vi "Settings Dialog.vi"(8 "error in (no error)":errorcluster, 11 "Feed Module Config in":T18={"GUID"="", "Drop Coords"={"Horizontal"=0, "Vertical"=0}, "Process Name"="", "Queue Name"="", "Settings"={"Cycle Period"=500.0, "Ismatech"={"VISA resource name"="", "Simulated?"=TRUE, "Pump Number"=1.0, "Reverse?"=FALSE}, "Masterflex"={"VISA resource name"="", "Simulated?"=TRUE, "Pump Number"=1.0, "Reverse?"=FALSE}, "Mettler"={"VISA resource name"="", "Simulated?"=FALSE}, "Bronkhorst M13 Flow Meter"={"VISA resource name"="", "Simulated?"=TRUE, "Smoothing Steps"=1}, "PID 2 Parameters"={"Input Device"=enum."Default", "Output Device"=enum."Default", "Setpoint"=0.0, "PID gains"={"proportional gain (Kc)"=1.0, "integral time (Ti, min)"=0.01, "derivative time (Td, min)"=0.0}}, "Manual Entry"=0.0, "Auto?"=TRUE, "output range"={"output high"=100.0, "output low"=0.0}, "Tacmina Settings"={"Analog DAQ Task"="", "Digital DAQ Task"=""}, "KNF SIMDOS Settings"={"VISA resource name"="", "Simulated?"=TRUE}, "ASIA Pump C"={"ASIA Pump #"=-1, "channel"=-1, "Simulated"=FALSE}, "VICI Settings"={"VISA resource name"="", "Simulated?"=TRUE, "Pump Letter"="", "Reverse?"=FALSE}, "FLOM Settings"={"VISA resource name"="", "Simulated?"=TRUE, "Pump Number"=0.0}, "SSI PR/LD Settings"={"VISA resource name"="", "Simulated?"=FALSE}, "Masterflex 75211 Settings"={"Analog DAQ Task"="", "Digital DAQ Task"=""}, "SSI P40 Settings"={"VISA resource name"="", "Simulated?"=TRUE}, "Ismatech 3 Channel Settings"={"VISA resource name"="", "Pump Number"=1, "Channel Number"=0, "Simulated?"=TRUE, "Reverse?"=FALSE}, "Bronkhorst M14 Settings"={"VISA resource name"="", "Simulated?"=FALSE, "Smoothing Steps"=1}}, "Settings Load Count"=0, "OP Load Count"=0} {"Settings"."Bronkhorst M14 Settings"."Smoothing Steps" min=1 step=1; "Settings"."Ismatech 3 Channel Settings"."Channel Number" min=0 max=3; "Settings"."Ismatech 3 Channel Settings"."Pump Number" min=1; "Settings"."output range"."output low" min=0.0 max=100.0 format="%.2f"; "Settings"."output range"."output high" format="%.2f"; "Settings"."PID 2 Parameters"."PID gains"."derivative time (Td, min)" format="%.3f"; "Settings"."PID 2 Parameters"."PID gains"."integral time (Ti, min)" format="%.3f"; "Settings"."PID 2 Parameters"."PID gains"."proportional gain (Kc)" format="%.3f"; "Settings"."Bronkhorst M13 Flow Meter"."Smoothing Steps" min=1 step=1; "Settings"."ASIA Pump C"."channel" min=0 max=1 step=1; "Settings"."Ismatech"."Pump Number" min=1.0 max=20.0 step=1.0; "Settings"."Masterflex"."Pump Number" min=1.0 max=20.0 step=1.0}) -> (0 "error out":errorcluster, 1 "Cancelled?":bool=TRUE, 2 "UI Refresh Needed?":bool, 3 "Feed Module Config out":T18={"GUID"="", "Drop Coords"={"Horizontal"=0, "Vertical"=0}, "Process Name"="", "Queue Name"="", "Settings"={"Cycle Period"=500.0, "Ismatech"={"VISA resource name"="", "Simulated?"=TRUE, "Pump Number"=1.0, "Reverse?"=FALSE}, "Masterflex"={"VISA resource name"="", "Simulated?"=TRUE, "Pump Number"=1.0, "Reverse?"=FALSE}, "Mettler"={"VISA resource name"="", "Simulated?"=FALSE}, "Bronkhorst M13 Flow Meter"={"VISA resource name"="", "Simulated?"=TRUE, "Smoothing Steps"=1}, "PID 2 Parameters"={"Input Device"=enum."Default", "Output Device"=enum."Default", "Setpoint"=0.0, "PID gains"={"proportional gain (Kc)"=1.0, "integral time (Ti, min)"=0.01, "derivative time (Td, min)"=0.0}}, "Manual Entry"=0.0, "Auto?"=TRUE, "output range"={"output high"=100.0, "output low"=0.0}, "Tacmina Settings"={"Analog DAQ Task"="", "Digital DAQ Task"=""}, "KNF SIMDOS Settings"={"VISA resource name"="", "Simulated?"=TRUE}, "ASIA Pump C"={"ASIA Pump #"=0, "channel"=0, "Simulated"=FALSE}, "VICI Settings"={"VISA resource name"="", "Simulated?"=TRUE, "Pump Letter"="", "Reverse?"=FALSE}, "FLOM Settings"={"VISA resource name"="", "Simulated?"=TRUE, "Pump Number"=0.0}, "SSI PR/LD Settings"={"VISA resource name"="", "Simulated?"=FALSE}, "Masterflex 75211 Settings"={"Analog DAQ Task"="", "Digital DAQ Task"=""}, "SSI P40 Settings"={"VISA resource name"="", "Simulated?"=TRUE}, "Ismatech 3 Channel Settings"={"VISA resource name"="", "Pump Number"=1, "Channel Number"=0, "Simulated?"=TRUE, "Reverse?"=FALSE}, "Bronkhorst M14 Settings"={"VISA resource name"="", "Simulated?"=FALSE, "Smoothing Steps"=1}}, "Settings Load Count"=0, "OP Load Count"=0} {"Settings"."Bronkhorst M14 Settings"."Smoothing Steps" min=1 step=1; "Settings"."Ismatech 3 Channel Settings"."Channel Number" min=0 max=3; "Settings"."Ismatech 3 Channel Settings"."Pump Number" min=1; "Settings"."output range"."output low" min=0.0 max=100.0 format="%.2f"; "Settings"."output range"."output high" format="%.2f"; "Settings"."PID 2 Parameters"."PID gains"."derivative time (Td, min)" format="%.3f"; "Settings"."PID 2 Parameters"."PID gains"."integral time (Ti, min)" format="%.3f"; "Settings"."PID 2 Parameters"."PID gains"."proportional gain (Kc)" format="%.3f"; "Settings"."Bronkhorst M13 Flow Meter"."Smoothing Steps" min=1 step=1; "Settings"."ASIA Pump C"."channel" min=0 max=1 step=1; "Settings"."Ismatech"."Pump Number" min=1.0 max=20.0 step=1.0; "Settings"."Masterflex"."Pump Number" min=1.0 max=20.0 step=1.0})   [LabVIEW 2018, in "Feed Module.lvlib" / "Settings.lvlib"]
doc: "Dialog for selecting user specified settings."
uses:
  Settings.lvlib
  Feed Module/Controls/Feed Module Config Cluster.ctl
  <vilib>/Utility/miscctls.llb/LVPoint32TypeDef.ctl
  Feed Module/Controls/Feed Module Settings Cluster.ctl
  Ismatec ISM 831C/Controls/Ismatech ISM831C Settings Cluster.ctl
  Masterflex 7550-30/Controls/Settings Cluster.ctl
  Mettler Toledo/Controls/Settings Cluster.ctl
  Bronkhorst M13 Flow Meter/Settings Cluster.ctl
  Measure Instrument/PID 2 Parameters Cluster.ctl
  Measure Instrument/PID Input Enum.ctl
  Measure Instrument/PID 2 Output Enum.ctl
  Tacmina QI/Tacmina QI DAQ Setting.ctl
  KNF Pump/Settings Cluster plus SIMDOS.ctl
  ASIA Pump/Pump Settings.ctl
  VICI M50 Party Mode/Settings Cluster.ctl
  FLOM Pump/Settings Cluster.ctl
  SSI PR Class/SSI PR or LD Settings Cluster.ctl
  Masterflex 75211/Masterflex 75211 DAQ Setting.ctl
  SSI PR Class/SSI P40 Settings Cluster.ctl
  Ismatec 78001/Ismatec 4083.ctl
  Bronkhorst M14 Flow Meter/Settings Cluster.ctl
  Ismatec ISM 831C/Ismatec ISM 831C.lvlib
  Masterflex 7550-30/Masterflex 7550-30.lvlib
  Mettler Toledo/Mettler Toledo.lvlib
  Bronkhorst M13 Flow Meter/Bronkhorst M13 Flow Meter.lvlib
  Bronkhorst M14 Flow Meter/Bronkhorst M14 Flow Meter.lvlib
  KNF Pump/KNF SIMDOS.lvlib
  VICI M50 Party Mode/VICI M6 M50 Party Mode.lvlib
  FLOM Pump/FLOM Pump.lvlib
  ASIA Pump.lvlib
  SSI PR Class/SSI PR or LD Pump.lvlib
  SSI PR Class/SSI P40 Pump.lvlib
  Ismatec 78001/Ismatec 4308.lvlib
  Feed Module/Feed Module.lvlib
  Tacmina QI/Tacmina QI.lvlib
  Masterflex 75211/Masterflex 75211.lvlib
panel:
  in  "Module Name":string
  in  "Settings Dialog":T17={"Cycle Period"=500.0, "Ismatech"={"VISA resource name"="", "Simulated?"=FALSE, "Pump Number"=1.0, "Reverse?"=FALSE}, "Masterflex"={"VISA resource name"="", "Simulated?"=FALSE, "Pump Number"=1.0, "Reverse?"=FALSE}, "Mettler"={"VISA resource name"="", "Simulated?"=FALSE}, "Bronkhorst M13 Settings"={"VISA resource name"="", "Simulated?"=FALSE, "Smoothing Steps"=1}, "PID 2 Parameters"={"Input Device"=enum."Default", "Output Device"=enum."Default", "PID gains"={"proportional gain (Kc)"=1.0, "integral time (Ti, min)"=0.01, "derivative time (Td, min)"=0.0}}, "PID2 Range"={"output high"=100.0, "output low"=0.0}, "Bronkhorst M14 Settings"={"VISA resource name"="", "Simulated?"=FALSE, "Smoothing Steps"=1}, "Tacmina Settings"={"Analog DAQ Task"="", "Digital DAQ Task"=""}, "KNF SIMDOS Settings"={"VISA resource name"="", "Simulated?"=FALSE}, "ASIA Pump C"={"ASIA Pump #"=-1, "channel"=-1, "Simulated"=FALSE}, "VICI M50 Settings"={"VISA resource name"="", "Simulated?"=FALSE, "Pump Letter"="", "Reverse?"=FALSE}, "FLOM Settings"={"VISA resource name"="", "Simulated?"=FALSE, "Pump Number"=1.0}, "SSI PR/LD Settings"={"VISA resource name"="", "Simulated?"=FALSE}, "Masterflex 75211 Settings"={"Analog DAQ Task"="", "Digital DAQ Task"=""}, "SSI P40 Settings"={"VISA resource name"="", "Simulated?"=FALSE}, "Ismatech 3 Channel Settings"={"VISA resource name"="", "Pump Number"=0, "Channel Number"=0, "Simulated?"=FALSE, "Reverse?"=FALSE}} {"Ismatech 3 Channel Settings"."Channel Number" min=0 max=3; "Ismatech 3 Channel Settings"."Pump Number" min=1; "ASIA Pump C"."channel" min=-1 max=1 step=1; "Bronkhorst M14 Settings"."Smoothing Steps" min=1 step=1; "PID2 Range"."output low" min=0.0 max=100.0 format="%.2f"; "PID2 Range"."output high" format="%.2f"; "PID 2 Parameters"."PID gains"."derivative time (Td, min)" format="%.3f"; "PID 2 Parameters"."PID gains"."integral time (Ti, min)" format="%.3f"; "PID 2 Parameters"."PID gains"."proportional gain (Kc)" format="%.3f"; "Bronkhorst M13 Settings"."Smoothing Steps" min=1 step=1; "Masterflex"."Pump Number" min=1.0 max=20.0 step=1.0; "Ismatech"."Pump Number" min=1.0 max=20.0 step=1.0}
  in  "Cancel Button":bool
  in  "OK Button":bool
  # "Non visible portion of dialog (needed for connector pane)."
  # "Output Instruments"
  # "Input Instruments"
  # "Output Instruments"
  # "Input Instruments"
  # "Output Instruments"
  # "Input Instruments"
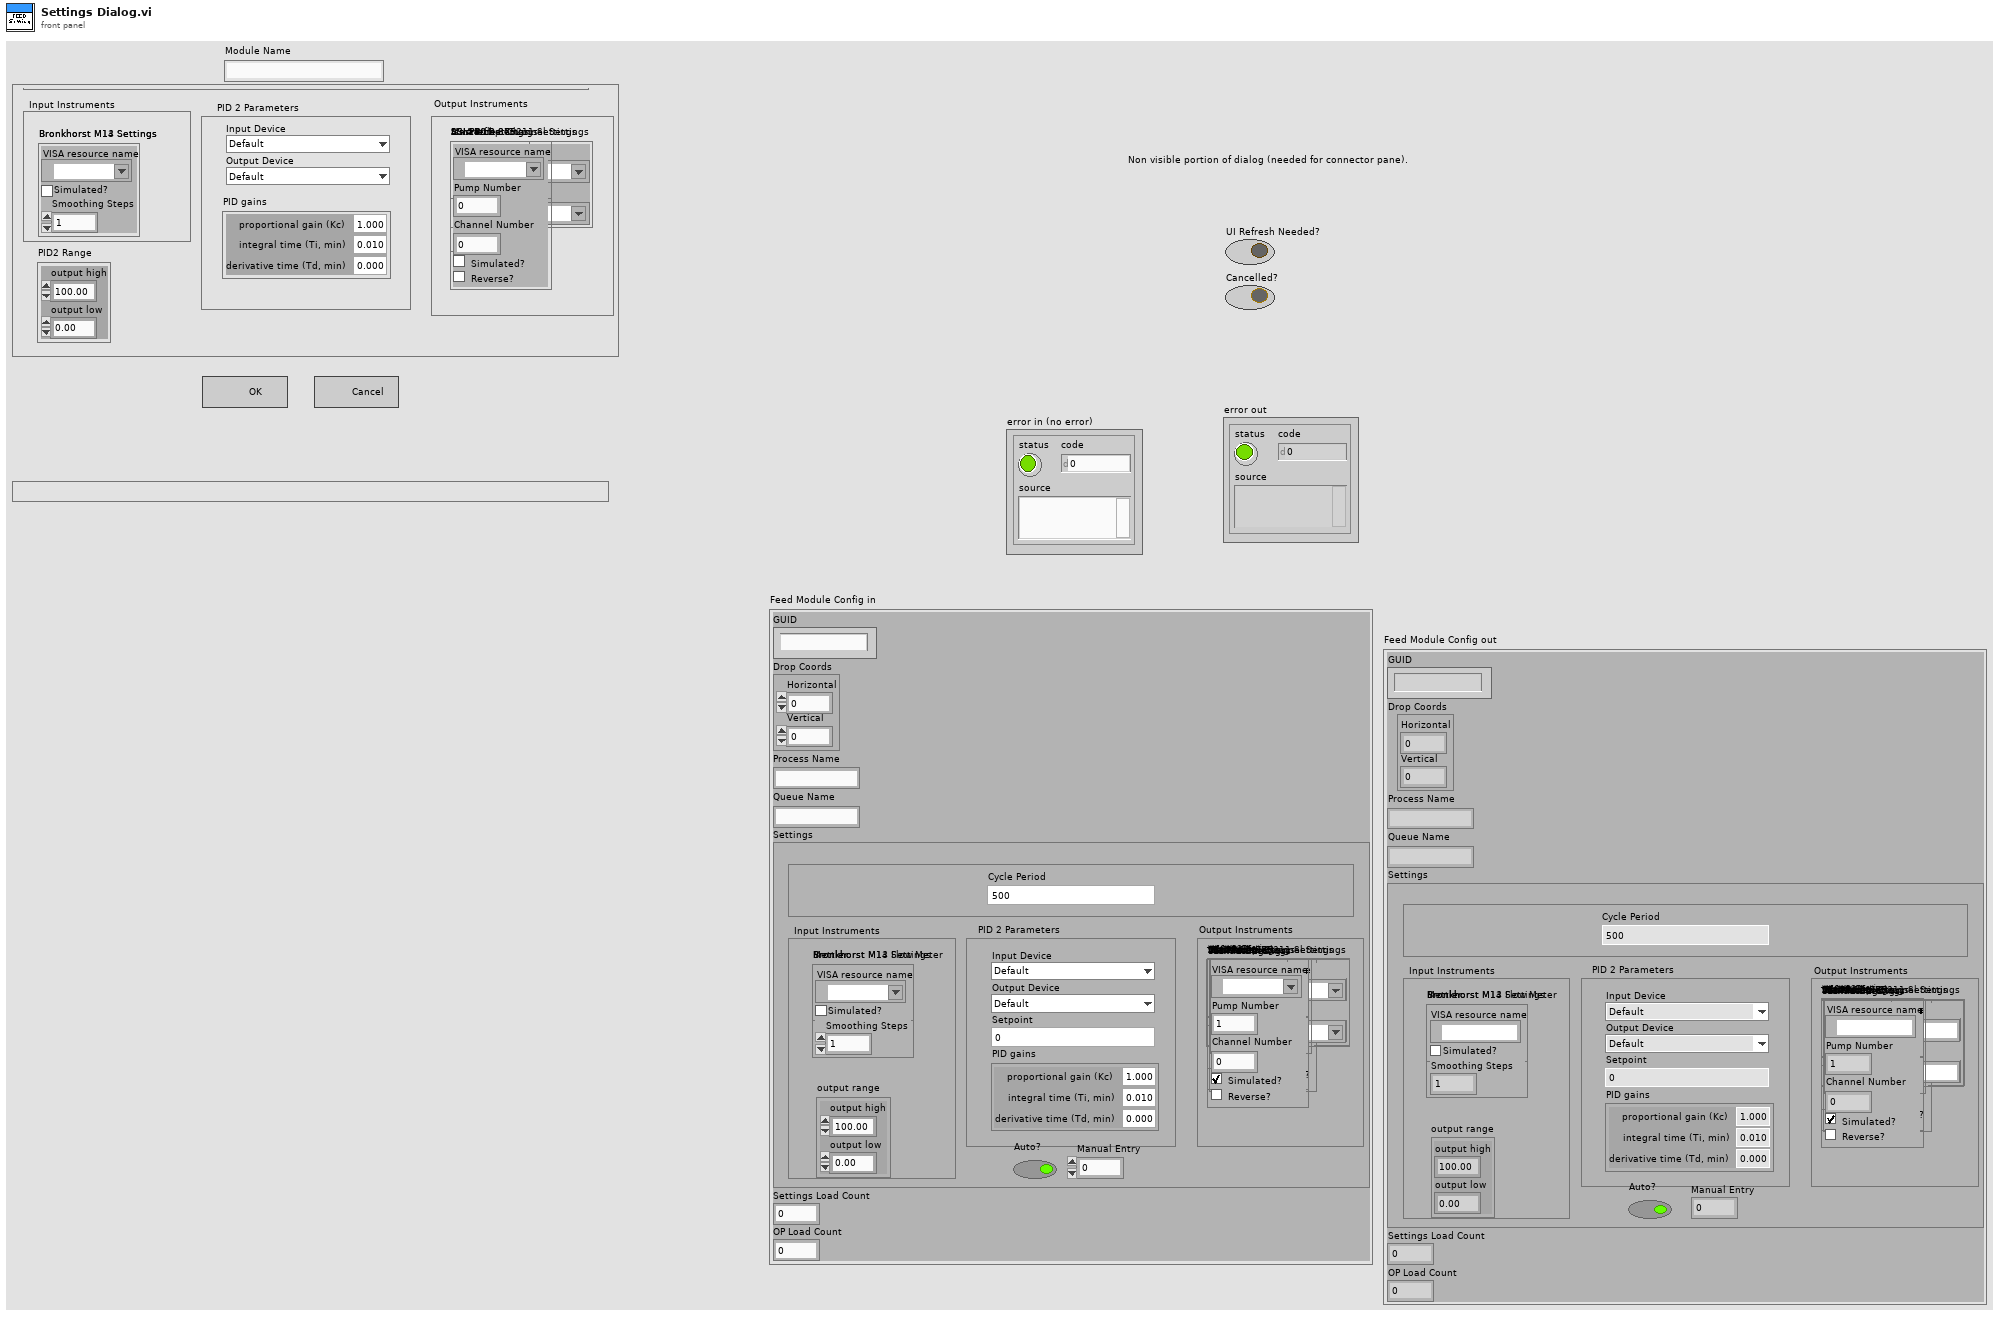
[diagram p1: front panel]
types:
  T1 = typedef "Ismatec ISM 831C.lvlib/Ismatech ISM831C Settings Cluster.ctl" = cluster{"VISA resource name":refnum<visa-resource-name>, "Simulated?":bool, "Pump Number":dbl, "Reverse?":bool}
  T2 = typedef "Masterflex 7550-30.lvlib/Settings Cluster.ctl" = cluster{"VISA resource name":refnum<visa-resource-name>, "Simulated?":bool, "Pump Number":dbl, "Reverse?":bool}
  T3 = typedef "Mettler Toledo.lvlib/Settings Cluster.ctl" = cluster{"VISA resource name":refnum<visa-resource-name>, "Simulated?":bool}
  T4 = typedef "Bronkhorst M13 Flow Meter.lvlib/Settings Cluster.ctl" = cluster{"VISA resource name":refnum<visa-resource-name>, "Simulated?":bool, "Smoothing Steps":i32}
  T5 = typedef "PID Input Enum.ctl" = enum16{"Default", "Bronkhorst M13", "Bronkhorst M14", "Scale Rate of Change"}
  T6 = typedef "PID 2 Output Enum.ctl" = enum16{"Default", "Ismatec ISM 4308", "Ismatec ISM 831C", "Masterflex 7550-30", "VICI", "Tacmina QI", "KNF SIMDOS", "ASIA Type C", "FLOM UI-22-11", "SSI PR/LD", "SSI P40", "Masterflex 75211-70"}
  T7 = typedef "Bronkhorst M14 Flow Meter.lvlib/Settings Cluster.ctl" = cluster{"VISA resource name":refnum<visa-resource-name>, "Simulated?":bool, "Smoothing Steps":i32}
  T8 = typedef "Tacmina QI.lvlib/Tacmina QI DAQ Setting.ctl" = cluster{"Analog DAQ Task":refnum<k21>, "Digital DAQ Task":refnum<k21>}
  T9 = typedef "KNF SIMDOS.lvlib/Settings Cluster plus SIMDOS.ctl" = cluster{"VISA resource name":refnum<visa-resource-name>, "Simulated?":bool}
  T10 = typedef "ASIA Pump.lvlib/Pump Settings.ctl" = cluster{"ASIA Pump #":i32, "channel":i32, "Simulated":bool}
  T11 = typedef "VICI M6 M50 Party Mode.lvlib/Settings Cluster.ctl" = cluster{"VISA resource name":refnum<visa-resource-name>, "Simulated?":bool, "Pump Letter":string, "Reverse?":bool}
  T12 = typedef "FLOM Pump.lvlib/Settings Cluster.ctl" = cluster{"VISA resource name":refnum<visa-resource-name>, "Simulated?":bool, "Pump Number":dbl}
  T13 = typedef "SSI PR or LD Pump.lvlib/SSI PR or LD Settings Cluster.ctl" = cluster{"VISA resource name":refnum<visa-resource-name>, "Simulated?":bool}
  T14 = typedef "Masterflex 75211.lvlib/Masterflex 75211 DAQ Setting.ctl" = cluster{"Analog DAQ Task":refnum<k21>, "Digital DAQ Task":refnum<k21>}
  T15 = typedef "SSI P40 Pump.lvlib/SSI P40 Settings Cluster.ctl" = cluster{"VISA resource name":refnum<visa-resource-name>, "Simulated?":bool}
  T16 = typedef "Ismatec 4308.lvlib/Ismatec 4083.ctl" = cluster{"VISA resource name":refnum<visa-resource-name>, "Pump Number":i16, "Channel Number":i16, "Simulated?":bool, "Reverse?":bool}
  T17 = cluster{"Cycle Period":dbl, "Ismatech":T1, "Masterflex":T2, "Mettler":T3, "Bronkhorst M13 Settings":T4, "PID 2 Parameters":cluster{"Input Device":T5, "Output Device":T6, "PID gains":cluster{"proportional gain (Kc)":dbl, "integral time (Ti, min)":dbl, "derivative time (Td, min)":dbl}}, "PID2 Range":cluster{"output high":dbl, "output low":dbl}, "Bronkhorst M14 Settings":T7, "Tacmina Settings":T8, "KNF SIMDOS Settings":T9, "ASIA Pump C":T10, "VICI M50 Settings":T11, "FLOM Settings":T12, "SSI PR/LD Settings":T13, "Masterflex 75211 Settings":T14, "SSI P40 Settings":T15, "Ismatech 3 Channel Settings":T16}
  T18 = typedef "Feed Module.lvlib/Feed Module Config Cluster.ctl" = cluster{"GUID":string, "Drop Coords":T19, "Process Name":string, "Queue Name":string, "Settings":T20, "Settings Load Count":i32, "OP Load Count":i32}
  T19 = typedef "LVPoint32TypeDef.ctl" = cluster{"Horizontal":i32, "Vertical":i32}
  T20 = typedef "Feed Module.lvlib/Feed Module Settings Cluster.ctl" = cluster{"Cycle Period":dbl, "Ismatech":T1, "Masterflex":T2, "Mettler":T3, "Bronkhorst M13 Flow Meter":T4, "PID 2 Parameters":T21, "Manual Entry":dbl, "Auto?":bool, "output range":cluster{"output high":dbl, "output low":dbl}, "Tacmina Settings":T8, "KNF SIMDOS Settings":T9, "ASIA Pump C":T10, "VICI Settings":T11, "FLOM Settings":T12, "SSI PR/LD Settings":T13, "Masterflex 75211 Settings":T14, "SSI P40 Settings":T15, "Ismatech 3 Channel Settings":T16, "Bronkhorst M14 Settings":T7}
  T21 = typedef "PID 2 Parameters Cluster.ctl" = cluster{"Input Device":T5, "Output Device":T6, "Setpoint":dbl, "PID gains":cluster{"proportional gain (Kc)":dbl, "integral time (Ti, min)":dbl, "derivative time (Td, min)":dbl}}
  T22 = enum8{"Enabled", "Disabled", "Disabled and Grayed Out"}
  T23 = cluster{"Input Device":T5, "Output Device":T6, "PID gains":cluster{"proportional gain (Kc)":dbl, "integral time (Ti, min)":dbl, "derivative time (Td, min)":dbl}}
  T24 = cluster{"proportional gain (Kc)":dbl, "integral time (Ti, min)":dbl, "derivative time (Td, min)":dbl}
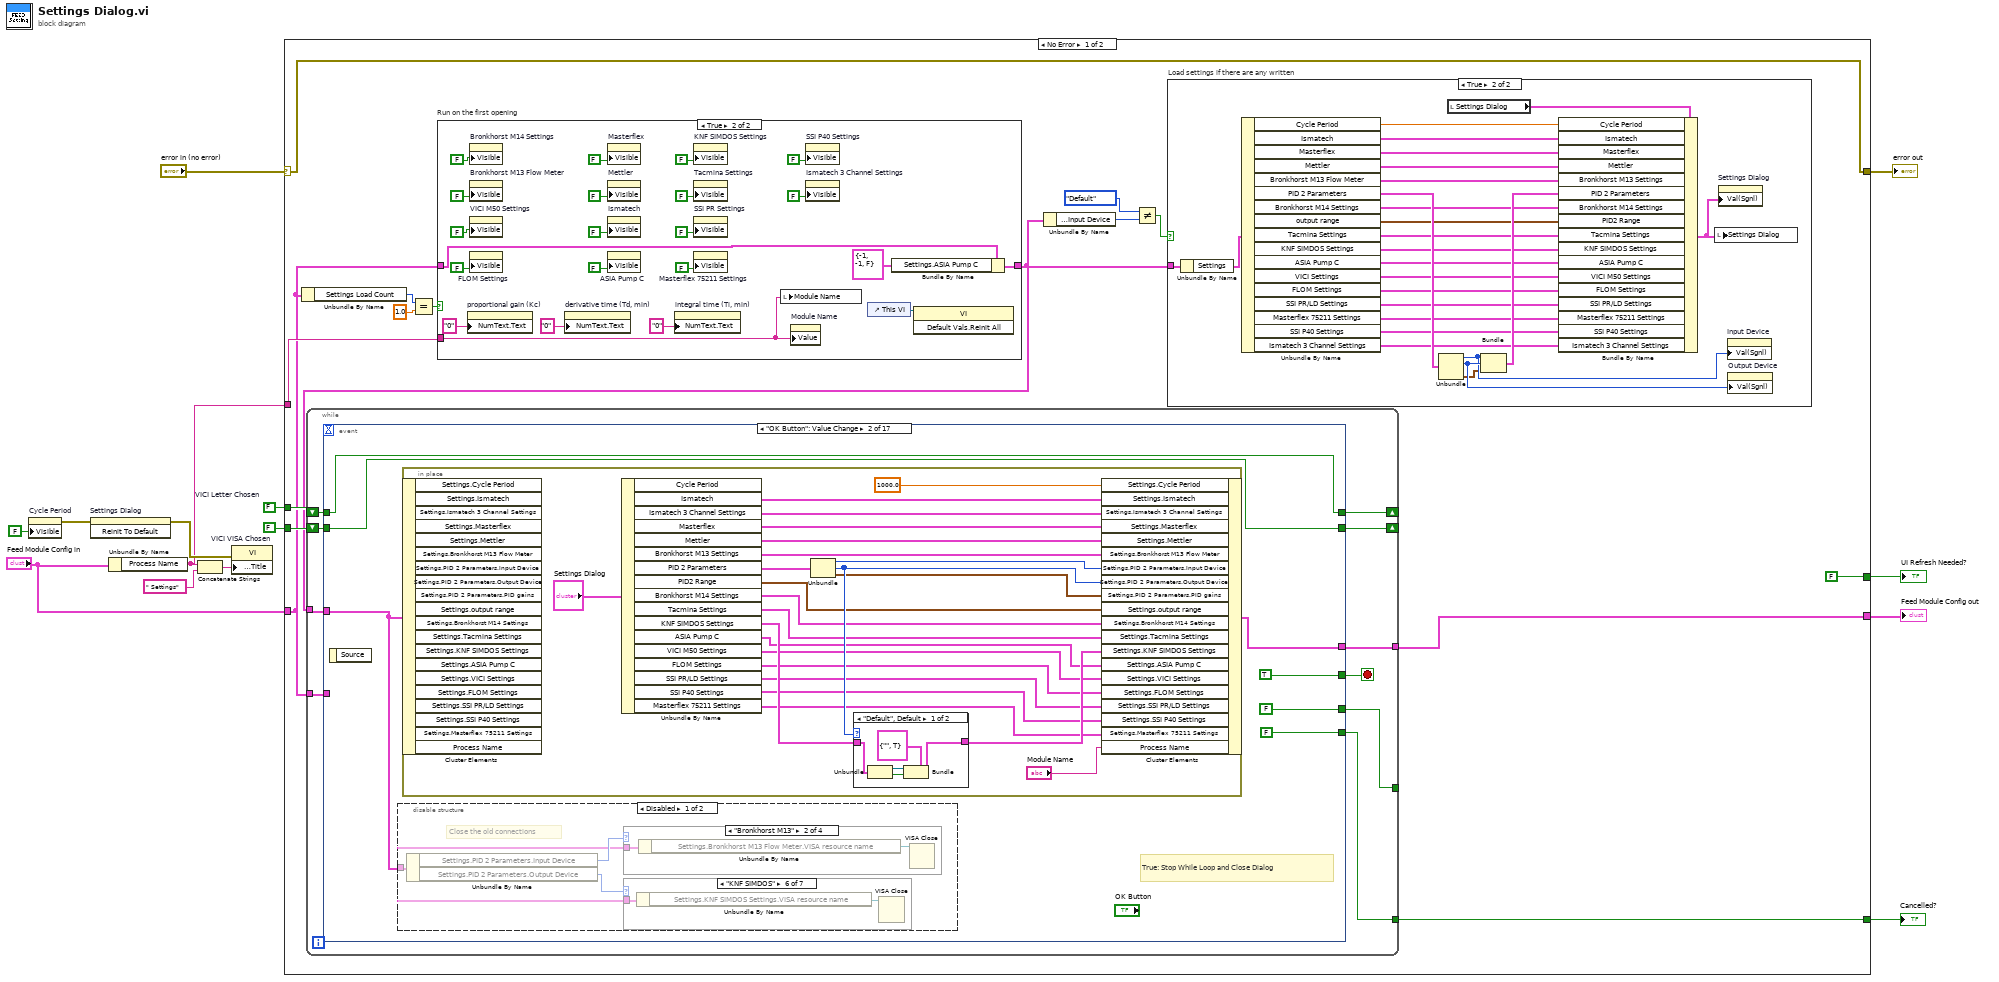
[diagram p0: block diagram]
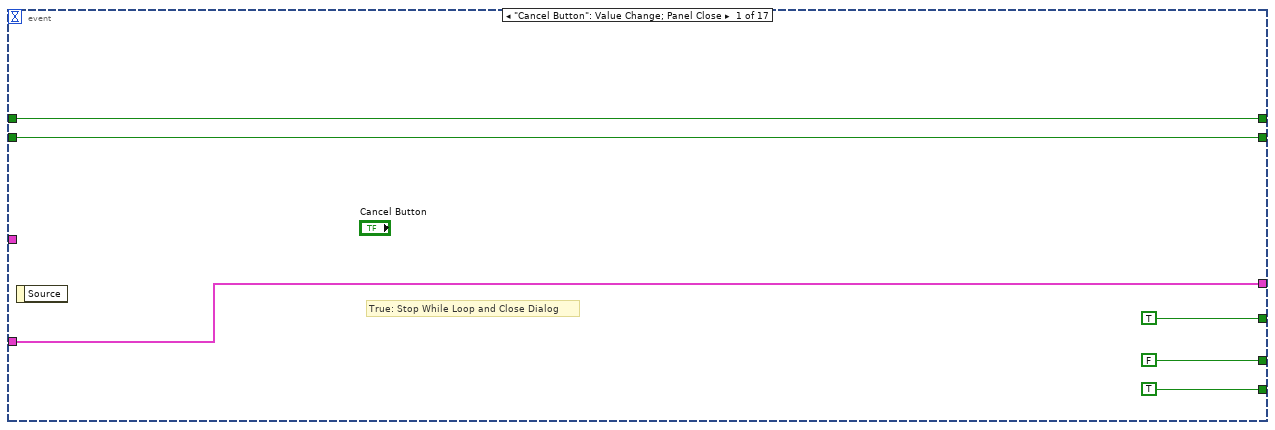
[diagram p4: hidden frame]
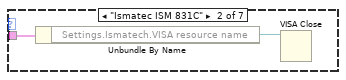
[diagram p6: hidden frame]
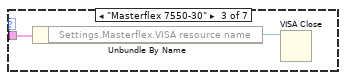
[diagram p7: hidden frame]
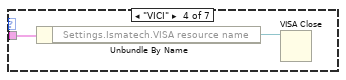
[diagram p8: hidden frame]
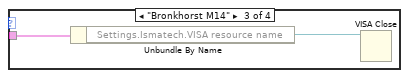
[diagram p12: hidden frame]
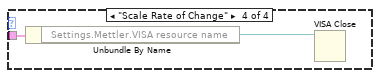
[diagram p13: hidden frame]
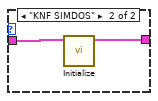
[diagram p15: hidden frame]
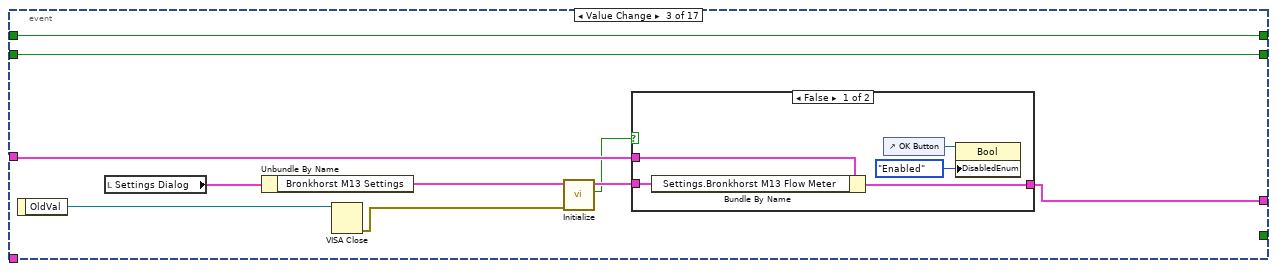
[diagram p16: hidden frame]
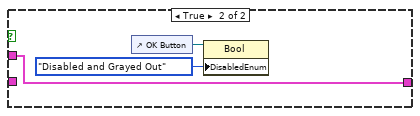
[diagram p17: hidden frame]
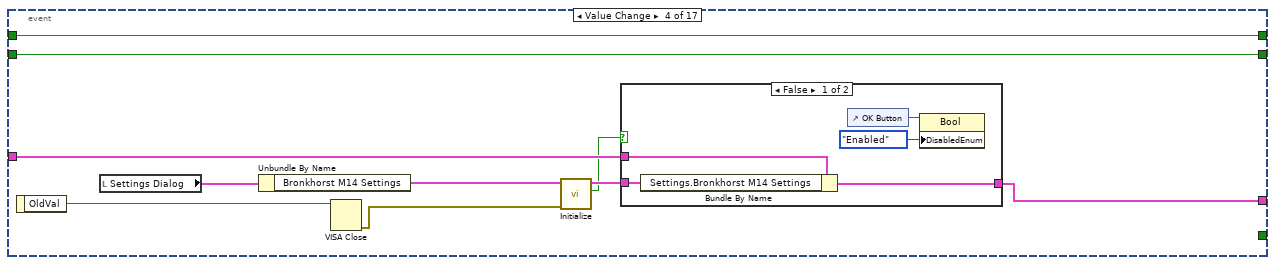
[diagram p18: hidden frame]
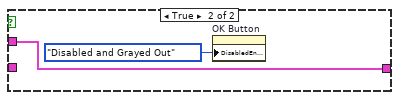
[diagram p19: hidden frame]
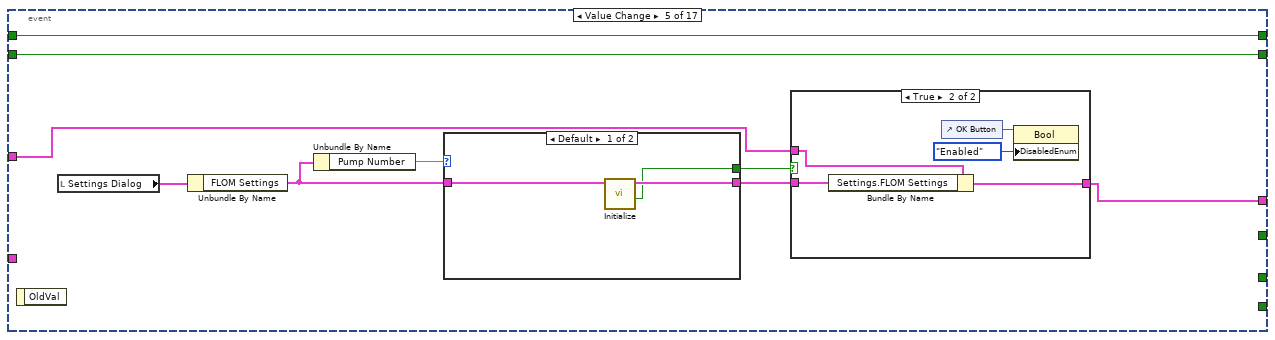
[diagram p20: hidden frame]
diagram:
  w5 = FALSE  # VICI VISA Chosen
  w6 = FALSE  # VICI Letter Chosen
  n1 = property on="Cycle Period" class="DigNum (strict)"("Visible"=FALSE) -> (error out=w3:errorcluster)  [unwired: 2 in, 1 out]
  n2 = invoke on="Settings Dialog" class="Clust (strict)" method="Reinit To Default"(error in=w3) -> (error out=w2:errorcluster)  [unwired: 2 in, 2 out]
  n3 = Unbundle By Name("Feed Module Config in") -> ("Process Name"=w1:string)
  n4 = Concatenate Strings(w1, " Settings" ("string")) -> (w8:string)
  n5 = property class="VI"(error in=w2, "Front Panel.Title"=w8) -> ()  [unwired: 1 in, 2 out]
  n6 = case shown="No Error" "error in (no error)" {
    selector: "error in (no error)" -> [w29 w630]
    tunnel: [w29 w630] -> w14
    tunnel: "Feed Module Config in" -> [w15 w629]
    tunnel: [w27 w629] -> w10
    tunnel: [FALSE ("UI Refresh Needed?") _] -> w13
    tunnel: [w26 TRUE ("UI Refresh Needed?")] -> w12
    tunnel: w6 -> [w22 _]
    tunnel: w5 -> [w21 _]
    tunnel: w1 -> [w20 _]
    frame No Error {
      n7 = Unbundle By Name(w15) -> ("Settings Load Count"=w25:i32)
      n8 = Equal?(x=w25, y=1.0) -> (x = y?=w23:bool)
      n9 = case "Run on the first opening" shown="True" w23 {
        tunnel: w15 -> [w55 w64]
        tunnel: [w55 w63] -> w19
        tunnel: w20 -> [_ w60]
        frame False {
        }
        frame True {
          n10 = property on="proportional gain (Kc)" class="DigNum (strict)"("NumText.Text"="0" ("Numeric Text.Text")) -> ()  [unwired: 2 in, 2 out]
          n11 = property on="Bronkhorst M14 Settings" class="Clust (strict)"("Visible"=FALSE) -> ()  [unwired: 2 in, 2 out]
          n12 = property on="Bronkhorst M13 Flow Meter" class="Clust (strict)"("Visible"=FALSE) -> ()  [unwired: 2 in, 2 out]
          n13 = property on="VICI M50 Settings" class="Clust (strict)"("Visible"=FALSE) -> ()  [unwired: 2 in, 2 out]
          n14 = property on="FLOM Settings" class="Clust (strict)"("Visible"=FALSE) -> ()  [unwired: 2 in, 2 out]
          n15 = property on="derivative time (Td, min)" class="DigNum (strict)"("NumText.Text"="0" ("Numeric Text.Text")) -> ()  [unwired: 2 in, 2 out]
          n16 = property on="Masterflex" class="Clust (strict)"("Visible"=FALSE) -> ()  [unwired: 2 in, 2 out]
          n17 = property on="Mettler" class="Clust (strict)"("Visible"=FALSE) -> ()  [unwired: 2 in, 2 out]
          n18 = property on="Ismatech" class="Clust (strict)"("Visible"=FALSE) -> ()  [unwired: 2 in, 2 out]
          n19 = property on="ASIA Pump C" class="Clust (strict)"("Visible"=FALSE) -> ()  [unwired: 2 in, 2 out]
          n20 = property on="integral time (Ti, min)" class="DigNum (strict)"("NumText.Text"="0" ("Numeric Text.Text")) -> ()  [unwired: 2 in, 2 out]
          n21 = property on="KNF SIMDOS Settings" class="Clust (strict)"("Visible"=FALSE) -> ()  [unwired: 2 in, 2 out]
          n22 = property on="Tacmina Settings" class="Clust (strict)"("Visible"=FALSE) -> ()  [unwired: 2 in, 2 out]
          n23 = property on="SSI PR Settings" class="Clust (strict)"("Visible"=FALSE) -> ()  [unwired: 2 in, 2 out]
          n24 = property on="Masterflex 75211 Settings" class="Clust (strict)"("Visible"=FALSE) -> ()  [unwired: 2 in, 2 out]
          n25 = local write "Module Name"(w60) -> ()
          n26 = property on="Module Name" class="Str"("Value"=w60) -> ()  [unwired: 2 in, 2 out]
          n27 = property on="SSI P40 Settings" class="Clust (strict)"("Visible"=FALSE) -> ()  [unwired: 2 in, 2 out]
          n28 = property on="Ismatech 3 Channel Settings" class="Clust (strict)"("Visible"=FALSE) -> ()  [unwired: 2 in, 2 out]
          n29 = control-ref of="This VI"() -> (w70:refnum<vi>)
          n30 = Bundle By Name(cluster=w64, "Settings.ASIA Pump C"=T10 {"ASIA Pump #"=-1, "channel"=-1, "Simulated"=FALSE}) -> (w63:T18)
          n31 = invoke class="VI" method="Default Vals.Reinit All"(reference=w70) -> ()  [unwired: 2 in, 3 out]
        }
      }
      n32 = while {
        tunnel: [w87] -> _
        tunnel: [w86] -> w27
        tunnel: [w84] -> w26
        shift-right: [w83] -> _
        shift-left: w22 -> [w82]
        shift-right: [w81] -> _
        shift-left: w21 -> [w80]
        tunnel: w19 -> [w79]
        tunnel: w15 -> [w78]
        stop <- w85 stop-if-true
        n33 = event shown="[1] \"OK Button\": Value Change" {
          selector: _ -> [_ _ _ _ _ _ _ _ _ _ _ _ _ _ _ _ _]
          dyn-events: _ -> [_ _ _ _ _ _ _ _ _ _ _ _ _ _ _ _ _]
          timeout: _ -> [_ _ _ _ _ _ _ _ _ _ _ _ _ _ _ _ _]
          tunnel: [w88 w94 w154 w172 w189 w215 w242 w253 w294 w311 w331 w345 w386 w552 w571 w588 w611] -> w86
          tunnel: w79 -> [_ w95 w153 w171 w190 w216 w241 w253 w295 w312 w332 w344 w386 w553 w572 w587 w610]
          tunnel: [FALSE ("UI Refresh Needed?") FALSE ("UI Refresh Needed?") _ _ _ _ _ _ _ _ _ _ _ _ _ _ _] -> w87
          tunnel: [TRUE TRUE _ _ _ _ _ _ _ _ _ _ _ _ _ _ _] -> w85
          tunnel: [TRUE ("UI Refresh Needed?") FALSE ("UI Refresh Needed?") _ _ _ _ _ _ _ _ _ _ _ _ _ _ _] -> w84
          tunnel: [w90 w97 w149 w167 w188 w213 w236 w260 w289 w308 w325 w343 w385 w550 w569 TRUE w604] -> w83
          tunnel: w82 -> [w90 w97 w149 w167 w188 w213 w236 w260 w289 w308 w325 w343 w385 w550 w569 _ w604]
          tunnel: [w89 w96 w148 w166 w187 w212 w235 w259 w288 w307 w324 w342 w384 w549 w568 w583 TRUE] -> w81
          tunnel: w80 -> [w89 w96 w148 w166 w187 w212 w235 w259 w288 w307 w324 w342 w384 w549 w568 w583 _]
          tunnel: w78 -> [w88 _ _ _ _ _ _ _ _ _ _ _ _ _ _ _ _]
          event "Cancel Button": Value Change; Panel Close {
            # "True: Stop While Loop and Close Dialog"
            n34 = event-data() -> ()  [unwired: 1 in, 1 out]
          }
          event "OK Button": Value Change {
            # "True: Stop While Loop and Close Dialog"
            n35 = event-data() -> ()  [unwired: 1 in, 1 out]
            n36 = disable-structure shown="Disabled" {
              disable-tunnel: w95 -> [w101 _]
              frame Disabled {
                # "Close the old connections"
                n37 = Unbundle By Name(w101) -> ("Settings.PID 2 Parameters.Input Device"=w103:T5, "Settings.PID 2 Parameters.Output Device"=w102:T6)
                n38 = case shown="\"Bronkhorst M13\"" w103 {
                  tunnel: w101 -> [_ w113 w114 w116]
                  frame "Default", Default {
                  }
                  frame "Bronkhorst M13" {
                    n39 = Unbundle By Name(w113) -> ("Settings.Bronkhorst M13 Flow Meter.VISA resource name"=w112:refnum<visa-resource-name>)
                    n40 = VISA Close(VISA resource name=w112) -> ()  [unwired: 1 in, 1 out]
                  }
                  frame "Bronkhorst M14" {
                    n41 = Unbundle By Name(w114) -> ("Settings.Ismatech.VISA resource name"=w115:refnum<visa-resource-name>)
                    n42 = VISA Close(VISA resource name=w115) -> ()  [unwired: 1 in, 1 out]
                  }
                  frame "Scale Rate of Change" {
                    n43 = Unbundle By Name(w116) -> ("Settings.Mettler.VISA resource name"=w117:refnum<visa-resource-name>)
                    n44 = VISA Close(VISA resource name=w117) -> ()  [unwired: 1 in, 1 out]
                  }
                }
                n45 = case shown="\"KNF SIMDOS\"" w102 {
                  tunnel: w101 -> [_ w104 w106 w108 _ w111 _]
                  frame "Default", Default {
                  }
                  frame "Ismatec ISM 831C" {
                    n46 = Unbundle By Name(w104) -> ("Settings.Ismatech.VISA resource name"=w105:refnum<visa-resource-name>)
                    n47 = VISA Close(VISA resource name=w105) -> ()  [unwired: 1 in, 1 out]
                  }
                  frame "Masterflex 7550-30" {
                    n48 = Unbundle By Name(w106) -> ("Settings.Masterflex.VISA resource name"=w107:refnum<visa-resource-name>)
                    n49 = VISA Close(VISA resource name=w107) -> ()  [unwired: 1 in, 1 out]
                  }
                  frame "VICI" {
                    n50 = Unbundle By Name(w108) -> ("Settings.Ismatech.VISA resource name"=w109:refnum<visa-resource-name>)
                    n51 = VISA Close(VISA resource name=w109) -> ()  [unwired: 1 in, 1 out]
                  }
                  frame "Tacmina QI" {
                    # "No VISA to Close"
                  }
                  frame "KNF SIMDOS" {
                    n52 = Unbundle By Name(w111) -> ("Settings.KNF SIMDOS Settings.VISA resource name"=w110:refnum<visa-resource-name>)
                    n53 = VISA Close(VISA resource name=w110) -> ()  [unwired: 1 in, 1 out]
                  }
                  frame "ASIA Type C" {
                    # "No VISA to Close"
                  }
                }
              }
              frame Enabled {
              }
            }
            n54 = in-place {
              n55 = in-place-cluster #1(w95) -> ()  [unwired: 20 out]
              n56 = Unbundle By Name("Settings Dialog") -> ("Ismatech"=w136:T1, "Ismatech 3 Channel Settings"=w119:T16, "Masterflex"=w135:T2, "Mettler"=w134:T3, "Bronkhorst M13 Settings"=w133:T4, "PID 2 Parameters"=w139:T23, "PID2 Range"=w129:cluster{"output high":dbl, "output low":dbl}, "Bronkhorst M14 Settings"=w118:T7, "Tacmina Settings"=w128:T8, "KNF SIMDOS Settings"=w138:T9, "ASIA Pump C"=w126:T10, "VICI M50 Settings"=w125:T11, "FLOM Settings"=w124:T12, "SSI PR/LD Settings"=w123:T13, "SSI P40 Settings"=w120:T15, "Masterflex 75211 Settings"=w121:T14)  [unwired: 1 out]
              n57 = Unbundle(w139) -> ("Input Device"=w132:T5, "Output Device"=w131:T6, "PID gains"=w130:T24)
              n58 = case shown="\"Default\", Default" w131 {
                tunnel: w138 -> [w145 w146]
                tunnel: [w144 w147] -> w127
                frame "Default", Default {
                  n59 = Unbundle(w145) -> ("VISA resource name"=w142:refnum<visa-resource-name>, "Simulated?"=w141:bool)
                  n60 = Bundle(cluster=T9 {"VISA resource name"="", "Simulated?"=TRUE} ("KNF Settings"), "VISA resource name"=w142, "Simulated?"=w141) -> (w144:T9)
                }
                frame "KNF SIMDOS" {
                  n61 = call "Initialize.vi"("KNF Settings In"=w146) -> ("KNF Settings Out"=w147:T9)  [unwired: 7 in, 3 out]
                }
              }
              n62 = in-place-cluster #1("Settings.Cycle Period"=1000.0, "Settings.Ismatech"=w136, "Settings.Ismatech 3 Channel Settings"=w119, "Settings.Masterflex"=w135, "Settings.Mettler"=w134, "Settings.Bronkhorst M13 Flow Meter"=w133, "Settings.PID 2 Parameters.Input Device"=w132, "Settings.PID 2 Parameters.Output Device"=w131, "Settings.PID 2 Parameters.PID gains"=w130, "Settings.output range"=w129, "Settings.Bronkhorst M14 Settings"=w118, "Settings.Tacmina Settings"=w128, "Settings.KNF SIMDOS Settings"=w127, "Settings.ASIA Pump C"=w126, "Settings.VICI Settings"=w125, "Settings.FLOM Settings"=w124, "Settings.SSI PR/LD Settings"=w123, "Settings.SSI P40 Settings"=w120, "Settings.Masterflex 75211 Settings"=w121, "Process Name"="Module Name") -> (w94:T18)
            }
          }
          event Value Change {
            n63 = event-data() -> ("OldVal"=w151:refnum<visa-resource-name>)  [unwired: 1 in]
            n64 = local read "Settings Dialog"() -> (w157:T17)
            n65 = Unbundle By Name(w157) -> ("Bronkhorst M13 Settings"=w156:T4)
            n66 = VISA Close(VISA resource name=w151) -> (error out=w152:errorcluster)  [unwired: 1 in]
            n67 = call "Initialize.vi"("error in (no error)"=w152, "Bronkhorst Settings in"=w156) -> ("No Meter Connnected"=w150:bool, "Bronkhorst Settings out"=w155:T4)  [unwired: 7 in, 1 out]
            n68 = case shown="False" w150 {
              tunnel: w155 -> [w162 _]
              tunnel: [w161 w165] -> w154
              tunnel: w153 -> [w160 w165]
              frame False {
                n69 = Bundle By Name(cluster=w160, "Settings.Bronkhorst M13 Flow Meter"=w162) -> (w161:T18)
                n70 = control-ref of="OK Button"() -> (w158:refnum<vi>)
                n71 = property on="Property Node" class="Bool"(reference=w158, "DisabledEnum"=T22."Enabled" ("Disabled")) -> ()  [unwired: 1 in, 2 out]
              }
              frame True {
                n72 = control-ref of="OK Button"() -> (w163:refnum<vi>)
                n73 = property on="Property Node" class="Bool"(reference=w163, "DisabledEnum"=T22."Disabled and Grayed Out" ("Disabled")) -> ()  [unwired: 1 in, 2 out]
              }
            }
          }
          event Value Change {
            n74 = event-data() -> ("OldVal"=w169:refnum<visa-resource-name>)  [unwired: 1 in]
            n75 = local read "Settings Dialog"() -> (w175:T17)
            n76 = Unbundle By Name(w175) -> ("Bronkhorst M14 Settings"=w174:T7)
            n77 = VISA Close(VISA resource name=w169) -> (error out=w170:errorcluster)  [unwired: 1 in]
            n78 = call "Initialize.vi"("error in (no error)"=w170, "Bronkhorst Settings in"=w174) -> ("No Meter Connected"=w168:bool, "Bronkhorst Settings out"=w173:T7)  [unwired: 7 in, 1 out]
            n79 = case shown="False" w168 {
              tunnel: w173 -> [w176 _]
              tunnel: [w180 w182] -> w172
              tunnel: w171 -> [w179 w182]
              frame False {
                n80 = Bundle By Name(cluster=w179, "Settings.Bronkhorst M14 Settings"=w176) -> (w180:T18)
                n81 = control-ref of="OK Button"() -> (w177:refnum<vi>)
                n82 = property on="Property Node" class="Bool"(reference=w177, "DisabledEnum"=T22."Enabled" ("Disabled")) -> ()  [unwired: 1 in, 2 out]
              }
              frame True {
                n83 = property on="OK Button" class="Bool"("DisabledEnum"=T22."Disabled and Grayed Out" ("Disabled")) -> ()  [unwired: 2 in, 2 out]
              }
            }
          }
          event Value Change {
            n84 = event-data() -> ()  [unwired: 1 in, 1 out]
            n85 = local read "Settings Dialog"() -> (w191:T17)
            n86 = Unbundle By Name(w191) -> ("FLOM Settings"=w184:T12)
            n87 = Unbundle By Name(w184) -> ("Pump Number"=w183:dbl)
            n88 = case shown="Default" w183 {
              tunnel: [w194 w197] -> w186
              tunnel: [w193 FALSE ("Initialized")] -> w185
              tunnel: w184 -> [w192 w197]
              frame Default {
                n89 = call "Initialize.vi"("FLOM Settings in"=w192) -> ("Initialized"=w193:bool, "FLOM Settings out"=w194:T12)  [unwired: 7 in, 2 out]
              }
              frame 0 {
                n90 = One Button Dialog(message="Choose a non-zero Pump Number") -> ()  [unwired: 1 in, 1 out]
              }
            }
            n91 = case shown="True" w185 {
              tunnel: w190 -> [w201 w206]
              tunnel: [w201 w205] -> w189
              tunnel: w186 -> [_ w204]
              frame False {
                n92 = control-ref of="OK Button"() -> (w199:refnum<vi>)
                n93 = property on="Property Node" class="Bool"(reference=w199, "DisabledEnum"=T22."Disabled and Grayed Out" ("Disabled")) -> ()  [unwired: 1 in, 2 out]
                n94 = One Button Dialog(message="No Pump Connected") -> ()  [unwired: 1 in, 1 out]
              }
              frame True {
                n95 = Bundle By Name(cluster=w206, "Settings.FLOM Settings"=w204) -> (w205:T18)
                n96 = control-ref of="OK Button"() -> (w202:refnum<vi>)
                n97 = property on="Property Node" class="Bool"(reference=w202, "DisabledEnum"=T22."Enabled" ("Disabled")) -> ()  [unwired: 1 in, 2 out]
              }
            }
          }
          event Value Change {
            n98 = event-data() -> ("OldVal"=w214:refnum<visa-resource-name>)  [unwired: 1 in]
            n99 = local read "Settings Dialog"() -> (w217:T17)
            n100 = Unbundle By Name(w217) -> ("FLOM Settings"=w208:T12)
            n101 = VISA Close(VISA resource name=w214) -> (error out=w211:errorcluster)  [unwired: 1 in]
            n102 = Unbundle By Name(w208) -> ("Pump Number"=w207:dbl)
            n103 = case shown="Default" w207 {
              tunnel: w211 -> [w221 _]
              tunnel: [w220 w224] -> w210
              tunnel: [w219 FALSE ("Initialized")] -> w209
              tunnel: w208 -> [w218 w224]
              frame Default {
                n104 = call "Initialize.vi"("error in (no error)"=w221, "FLOM Settings in"=w218) -> ("Initialized"=w219:bool, "FLOM Settings out"=w220:T12)  [unwired: 6 in, 2 out]
              }
              frame 0 {
                n105 = One Button Dialog(message="Choose a Pump Number") -> ()  [unwired: 1 in, 1 out]
              }
            }
            n106 = case shown="False" w209 {
              tunnel: w216 -> [w228 w233]
              tunnel: [w228 w232] -> w215
              tunnel: w210 -> [_ w231]
              frame False {
                n107 = control-ref of="OK Button"() -> (w226:refnum<vi>)
                n108 = One Button Dialog(message="No Pump Connected") -> ()  [unwired: 1 in, 1 out]
                n109 = property on="Property Node" class="Bool"(reference=w226, "DisabledEnum"=T22."Disabled and Grayed Out" ("Disabled")) -> ()  [unwired: 1 in, 2 out]
              }
              frame True {
                n110 = Bundle By Name(cluster=w233, "Settings.FLOM Settings"=w231) -> (w232:T18)
                n111 = control-ref of="OK Button"() -> (w229:refnum<vi>)
                n112 = property on="Property Node" class="Bool"(reference=w229, "DisabledEnum"=T22."Enabled" ("Disabled")) -> ()  [unwired: 1 in, 2 out]
              }
            }
          }
          event Value Change {
            n113 = event-data() -> ("OldVal"=w237:refnum<visa-resource-name>)  [unwired: 1 in]
            n114 = local read "Settings Dialog"() -> (w240:T17)
            n115 = Unbundle By Name(w240) -> ("Ismatech"=w239:T1)
            n116 = VISA Close(VISA resource name=w237) -> (error out=w238:errorcluster)  [unwired: 1 in]
            n117 = call "Initialize.vi"("error in (no error)"=w238, "Ismatech Settings"=w239) -> ("Initialized"=w234:bool, "Ismatech Settings"=w243:T1)  [unwired: 6 in, 2 out]
            n118 = case shown="False" w234 {
              tunnel: w243 -> [_ w252]
              tunnel: [w247 w251] -> w242
              tunnel: w241 -> [w247 w250]
              frame False {
                n119 = control-ref of="OK Button"() -> (w245:refnum<vi>)
                n120 = property on="Property Node" class="Bool"(reference=w245, "DisabledEnum"=T22."Disabled and Grayed Out" ("Disabled")) -> ()  [unwired: 1 in, 2 out]
                n121 = One Button Dialog(message="No Pump Connected") -> ()  [unwired: 1 in, 1 out]
              }
              frame True {
                n122 = Bundle By Name(cluster=w250, "Settings.Ismatech"=w252) -> (w251:T18)
                n123 = control-ref of="OK Button"() -> (w248:refnum<vi>)
                n124 = property on="Property Node" class="Bool"(reference=w248, "DisabledEnum"=T22."Enabled" ("Disabled")) -> ()  [unwired: 1 in, 2 out]
              }
            }
          }
          event Value Change {
            n125 = event-data() -> ("NewVal"=w254:T16)  [unwired: 1 in]
            n126 = Unbundle By Name(w254) -> ("VISA resource name"=w256:refnum<visa-resource-name>, "Pump Number"=w258:i16, "Channel Number"=w257:i16, "Simulated?"=w255:bool)
            n127 = case shown="False" w255 {
              tunnel: w258 -> [w262 _]
              tunnel: w257 -> [w261 _]
              tunnel: w256 -> [w269 _]
              tunnel: w254 -> [w263 _]
              frame False {
                n128 = Empty String/Path?(string/path=w269) -> (empty?=w268:bool)
                n129 = Greater Than 0?(x=w261) -> (x > 0?=w265:bool)
                n130 = Not(x=w268) -> (.not. x?=w267:bool)
                n131 = Greater Than 0?(x=w262) -> (x > 0?=w266:bool)
                n132 = Compound Arithmetic op=AND(w267, w266, w265) -> (w264:bool)
                n133 = case shown="True" w264 {
                  tunnel: w263 -> [_ w276]
                  tunnel: w262 -> [_ w273]
                  tunnel: w261 -> [_ w272]
                  frame False {
                    n134 = property on="OK Button" class="Bool"("DisabledEnum"=T22."Disabled and Grayed Out" ("Disabled")) -> ()  [unwired: 2 in, 2 out]
                  }
                  frame True {
                    n135 = call "Global Read.vi"("Pump Number"=w273) -> ("Initialized Channels"=w275:dbl[])  [unwired: 4 in, 6 out]
                    n136 = Search 1D Array(1D array=w275, element=w272) -> (index of element=w274:i32)  [unwired: 1 in]
                    n137 = Less Than 0?(x=w274) -> (x < 0?=w271:bool)
                    n138 = case shown="True" w271 {
                      tunnel: w276 -> [_ w282]
                      frame False {
                        n139 = One Button Dialog(message="This channel has already been initialized elsewhere") -> ()  [unwired: 1 in, 1 out]
                        n140 = property on="OK Button" class="Bool"("DisabledEnum"=T22."Disabled and Grayed Out" ("Disabled")) -> ()  [unwired: 2 in, 2 out]
                      }
                      frame True {
                        n141 = call "Initialize.vi"("Ismatech 3 Channel Settings In"=w282) -> ("error out"=w281:errorcluster, "No Pump Connected"=w280:bool)  [unwired: 7 in, 2 out]
                        n142 = case shown="False" w280 {
                          tunnel: [T22."Enabled" ("Disabled") T22."Disabled and Grayed Out" ("Disabled")] -> w279
                          frame False {
                          }
                          frame True {
                            n143 = One Button Dialog(message="No Pump Connected") -> ()  [unwired: 1 in, 1 out]
                          }
                        }
                        n144 = property on="OK Button" class="Bool"(error in=w281, "DisabledEnum"=w279) -> ()  [unwired: 1 in, 2 out]
                      }
                    }
                  }
                }
              }
              frame True {
                n145 = property on="OK Button" class="Bool"("DisabledEnum"=T22."Enabled" ("Disabled")) -> ()  [unwired: 2 in, 2 out]
              }
            }
          }
          event Value Change {
            n146 = event-data() -> ("OldVal"=w293:refnum<visa-resource-name>)  [unwired: 1 in]
            n147 = local read "Settings Dialog"() -> (w296:T17)
            n148 = Unbundle By Name(w296) -> ("KNF SIMDOS Settings"=w291:T9)
            n149 = VISA Close(VISA resource name=w293) -> (error out=w292:errorcluster)  [unwired: 1 in]
            n150 = call "Initialize.vi"("error in (no error)"=w292, "KNF Settings In"=w291) -> ("Initialized"=w287:bool, "KNF Settings Out"=w290:T9)  [unwired: 6 in, 2 out]
            n151 = case shown="False" w287 {
              tunnel: w295 -> [w300 w305]
              tunnel: [w300 w304] -> w294
              tunnel: w290 -> [_ w303]
              frame False {
                n152 = control-ref of="OK Button"() -> (w298:refnum<vi>)
                n153 = One Button Dialog(message="No Pump Connected") -> ()  [unwired: 1 in, 1 out]
                n154 = property on="Property Node" class="Bool"(reference=w298, "DisabledEnum"=T22."Disabled and Grayed Out" ("Disabled")) -> ()  [unwired: 1 in, 2 out]
              }
              frame True {
                n155 = Bundle By Name(cluster=w305, "Settings.KNF SIMDOS Settings"=w303) -> (w304:T18)
                n156 = control-ref of="OK Button"() -> (w301:refnum<vi>)
                n157 = property on="Property Node" class="Bool"(reference=w301, "DisabledEnum"=T22."Enabled" ("Disabled")) -> ()  [unwired: 1 in, 2 out]
              }
            }
          }
          event Value Change {
            n158 = event-data() -> ("OldVal"=w309:refnum<visa-resource-name>)  [unwired: 1 in]
            n159 = local read "Settings Dialog"() -> (w313:T17)
            n160 = Unbundle By Name(w313) -> ("Masterflex"=w315:T2)
            n161 = VISA Close(VISA resource name=w309) -> (error out=w310:errorcluster)  [unwired: 1 in]
            n162 = call "Initialize.vi"("error in (no error)"=w310, "Masterflex Settings in"=w315) -> ("Initialized"=w306:bool, "Masterflex Settings out"=w314:T2)  [unwired: 6 in, 2 out]
            n163 = case shown="False" w306 {
              tunnel: w314 -> [_ w319]
              tunnel: w312 -> [w318 w323]
              tunnel: [w318 w322] -> w311
              frame False {
                n164 = control-ref of="OK Button"() -> (w316:refnum<vi>)
                n165 = property on="Property Node" class="Bool"(reference=w316, "DisabledEnum"=T22."Disabled and Grayed Out" ("Disabled")) -> ()  [unwired: 1 in, 2 out]
              }
              frame True {
                n166 = Bundle By Name(cluster=w323, "Settings.Masterflex"=w319) -> (w322:T18)
                n167 = control-ref of="OK Button"() -> (w320:refnum<vi>)
                n168 = property on="Property Node" class="Bool"(reference=w320, "DisabledEnum"=T22."Enabled" ("Disabled")) -> ()  [unwired: 1 in, 2 out]
              }
            }
          }
          event Value Change {
            n169 = event-data() -> ("OldVal"=w328:refnum<visa-resource-name>)  [unwired: 1 in]
            n170 = local read "Settings Dialog"() -> (w333:T17)
            n171 = Unbundle By Name(w333) -> ("Mettler"=w330:T3)
            n172 = VISA Close(VISA resource name=w328) -> (error out=w327:errorcluster)  [unwired: 1 in]
            n173 = call "Initialize.vi"("error in (no error)"=w327, "Mettler Settings in"=w330) -> ("No Scale Connected"=w326:bool, "Mettler Settings out"=w329:T3)  [unwired: 7 in, 1 out]
            n174 = case shown="False" w326 {
              tunnel: w332 -> [w338 w341]
              tunnel: [w337 w341] -> w331
              tunnel: w329 -> [w336 _]
              frame False {
                n175 = Bundle By Name(cluster=w338, "Settings.Mettler"=w336) -> (w337:T18)
                n176 = control-ref of="OK Button"() -> (w334:refnum<vi>)
                n177 = property on="Property Node" class="Bool"(reference=w334, "DisabledEnum"=T22."Enabled" ("Disabled")) -> ()  [unwired: 1 in, 2 out]
              }
              frame True {
                n178 = control-ref of="OK Button"() -> (w339:refnum<vi>)
                n179 = property on="Property Node" class="Bool"(reference=w339, "DisabledEnum"=T22."Disabled and Grayed Out" ("Disabled")) -> ()  [unwired: 1 in, 2 out]
              }
            }
          }
          event Value Change {
            n180 = event-data() -> ("NewVal"=w346:T5)  [unwired: 1 in]
            n181 = case "Show the correct settings" shown="\"Bronkhorst M14\"" w346 {
              tunnel: [w348 w358 w368 w378] -> w345
              tunnel: w344 -> [w348 w358 w368 w378]
              frame "Bronkhorst M13" {
                n182 = Unbundle By Name(w348) -> ("Settings.Bronkhorst M13 Flow Meter.VISA resource name"=w350:refnum<visa-resource-name>)
                n183 = Unbundle By Name(w348) -> ("Settings.PID 2 Parameters.Input Device"=w349:T5)
                n184 = property on="Mettler" class="Clust (strict)"("Visible"=FALSE) -> ()  [unwired: 2 in, 2 out]
                n185 = property on="Bronkhorst M13 Flow Meter" class="Clust (strict)"("Visible"=TRUE) -> ()  [unwired: 2 in, 2 out]
                n186 = property on="Bronkhorst M14 Settings" class="Clust (strict)"("Visible"=FALSE) -> ()  [unwired: 2 in, 2 out]
                n187 = case shown="\"Default\", Default" w349 {
                  frame "Default", Default {
                    n188 = property on="derivative time (Td, min)" class="DigNum (strict)"("NumText.Text"="0" ("Numeric Text.Text")) -> ()  [unwired: 2 in, 2 out]
                    n189 = property on="proportional gain (Kc)" class="DigNum (strict)"("NumText.Text"=".4" ("Numeric Text.Text")) -> ()  [unwired: 2 in, 2 out]
                    n190 = property on="integral time (Ti, min)" class="DigNum (strict)"("NumText.Text"="0.035" ("Numeric Text.Text")) -> ()  [unwired: 2 in, 2 out]
                  }
                  frame "Bronkhorst M13".."Scale Rate of Change" {
                  }
                }
                n191 = control-ref of="VISA resource name"() -> (w351:refnum<vi>)
                n192 = property on="Property Node" class="VISAName"(reference=w351, "Value"=w350) -> ()  [unwired: 1 in, 2 out]
              }
              frame "Bronkhorst M14" {
                n193 = Unbundle By Name(w358) -> ("Settings.PID 2 Parameters.Input Device"=w359:T5)
                n194 = Unbundle By Name(w358) -> ("Settings.Ismatech.VISA resource name"=w360:refnum<visa-resource-name>)
                n195 = property on="Mettler" class="Clust (strict)"("Visible"=FALSE) -> ()  [unwired: 2 in, 2 out]
                n196 = property on="Bronkhorst M13 Flow Meter" class="Clust (strict)"("Visible"=FALSE) -> ()  [unwired: 2 in, 2 out]
                n197 = property on="Bronkhorst M14 Settings" class="Clust (strict)"("Visible"=TRUE) -> ()  [unwired: 2 in, 2 out]
                n198 = control-ref of="VISA resource name"() -> (w361:refnum<vi>)
                n199 = case shown="\"Default\", Default" w359 {
                  frame "Default", Default {
                    n200 = property on="derivative time (Td, min)" class="DigNum (strict)"("NumText.Text"="0" ("Numeric Text.Text")) -> ()  [unwired: 2 in, 2 out]
                    n201 = property on="proportional gain (Kc)" class="DigNum (strict)"("NumText.Text"=".4" ("Numeric Text.Text")) -> ()  [unwired: 2 in, 2 out]
                    n202 = property on="integral time (Ti, min)" class="DigNum (strict)"("NumText.Text"="0.035" ("Numeric Text.Text")) -> ()  [unwired: 2 in, 2 out]
                  }
                  frame "Bronkhorst M13".."Scale Rate of Change" {
                  }
                }
                n203 = property on="Property Node" class="VISAName"(reference=w361, "Value"=w360) -> ()  [unwired: 1 in, 2 out]
              }
              frame "Scale Rate of Change" {
                n204 = Unbundle By Name(w368) -> ("Settings.PID 2 Parameters.Input Device"=w369:T5)
                n205 = property on="Mettler" class="Clust (strict)"("Visible"=TRUE) -> ()  [unwired: 2 in, 2 out]
                n206 = property on="Bronkhorst M13 Flow Meter" class="Clust (strict)"("Visible"=FALSE) -> ()  [unwired: 2 in, 2 out]
                n207 = property on="Bronkhorst M14 Settings" class="Clust (strict)"("Visible"=FALSE) -> ()  [unwired: 2 in, 2 out]
                n208 = Unbundle By Name(w368) -> ("Settings.Mettler.VISA resource name"=w371:refnum<visa-resource-name>)
                n209 = control-ref of="VISA resource name"() -> (w370:refnum<vi>)
                n210 = case shown="\"Default\", Default" w369 {
                  frame "Default", Default {
                    n211 = property on="derivative time (Td, min)" class="DigNum (strict)"("NumText.Text"="0" ("Numeric Text.Text")) -> ()  [unwired: 2 in, 2 out]
                    n212 = property on="proportional gain (Kc)" class="DigNum (strict)"("NumText.Text"=".4" ("Numeric Text.Text")) -> ()  [unwired: 2 in, 2 out]
                    n213 = property on="integral time (Ti, min)" class="DigNum (strict)"("NumText.Text"="0.035" ("Numeric Text.Text")) -> ()  [unwired: 2 in, 2 out]
                  }
                  frame "Bronkhorst M13".."Scale Rate of Change" {
                  }
                }
                n214 = property on="Property Node" class="VISAName"(reference=w370, "Value"=w371) -> ()  [unwired: 1 in, 2 out]
              }
              frame "Default", Default {
                n215 = property on="Mettler" class="Clust (strict)"("Visible"=FALSE) -> ()  [unwired: 2 in, 2 out]
                n216 = property on="Bronkhorst M14 Settings" class="Clust (strict)"("Visible"=FALSE) -> ()  [unwired: 2 in, 2 out]
                n217 = property on="Bronkhorst M13 Flow Meter" class="Clust (strict)"("Visible"=FALSE) -> ()  [unwired: 2 in, 2 out]
                n218 = property on="proportional gain (Kc)" class="DigNum (strict)"("NumText.Text"="0" ("Numeric Text.Text")) -> ()  [unwired: 2 in, 2 out]
                n219 = property on="integral time (Ti, min)" class="DigNum (strict)"("NumText.Text"="0" ("Numeric Text.Text")) -> ()  [unwired: 2 in, 2 out]
                n220 = property on="derivative time (Td, min)" class="DigNum (strict)"("NumText.Text"="0" ("Numeric Text.Text")) -> ()  [unwired: 2 in, 2 out]
              }
            }
          }
          event Value Change {
            n221 = event-data() -> ("NewVal"=w387:T6)  [unwired: 1 in]
            n222 = case "Show the correct settings" shown="\"Ismatec ISM 4308\"" w387 {
              tunnel: w386 -> [w399 w413 w425 w441 w456 _ _ _ w501 w515 w528 w540]
              frame "Ismatec ISM 831C" {
                n223 = property on="Ismatech" class="Clust (strict)"("Visible"=TRUE) -> ()  [unwired: 2 in, 2 out]
                n224 = property on="KNF SIMDOS Settings" class="Clust (strict)"("Visible"=FALSE) -> ()  [unwired: 2 in, 2 out]
                n225 = property on="Tacmina Settings" class="Clust (strict)"("Visible"=FALSE) -> ()  [unwired: 2 in, 2 out]
                n226 = Unbundle By Name(w399) -> ("Settings.Ismatech.VISA resource name"=w400:refnum<visa-resource-name>)
                n227 = property on="VICI M50 Settings" class="Clust (strict)"("Visible"=FALSE) -> ()  [unwired: 2 in, 2 out]
                n228 = property on="Masterflex" class="Clust (strict)"("Visible"=FALSE) -> ()  [unwired: 2 in, 2 out]
                n229 = property on="ASIA Pump C" class="Clust (strict)"("Visible"=FALSE) -> ()  [unwired: 2 in, 2 out]
                n230 = control-ref of="VISA resource name"() -> (w401:refnum<vi>)
                n231 = property on="FLOM Settings" class="Clust (strict)"("Visible"=FALSE) -> ()  [unwired: 2 in, 2 out]
                n232 = property on="SSI PR Settings" class="Clust (strict)"("Visible"=FALSE) -> ()  [unwired: 2 in, 2 out]
                n233 = property on="Masterflex 75211 Settings" class="Clust (strict)"("Visible"=FALSE) -> ()  [unwired: 2 in, 2 out]
                n234 = property on="Property Node" class="VISAName"(reference=w401, "Value"=w400) -> ()  [unwired: 1 in, 2 out]
                n235 = property on="SSI P40 Settings" class="Clust (strict)"("Visible"=FALSE) -> ()  [unwired: 2 in, 2 out]
                n236 = property on="Ismatech 3 Channel Settings" class="Clust (strict)"("Visible"=FALSE) -> ()  [unwired: 2 in, 2 out]
              }
              frame "Ismatec ISM 4308" {
                n237 = property on="Ismatech" class="Clust (strict)"("Visible"=FALSE) -> ()  [unwired: 2 in, 2 out]
                n238 = property on="KNF SIMDOS Settings" class="Clust (strict)"("Visible"=FALSE) -> ()  [unwired: 2 in, 2 out]
                n239 = property on="Tacmina Settings" class="Clust (strict)"("Visible"=FALSE) -> ()  [unwired: 2 in, 2 out]
                n240 = Unbundle By Name(w413) -> ("Settings.Ismatech.VISA resource name"=w414:refnum<visa-resource-name>)
                n241 = property on="VICI M50 Settings" class="Clust (strict)"("Visible"=FALSE) -> ()  [unwired: 2 in, 2 out]
                n242 = property on="Masterflex" class="Clust (strict)"("Visible"=FALSE) -> ()  [unwired: 2 in, 2 out]
                n243 = property on="ASIA Pump C" class="Clust (strict)"("Visible"=FALSE) -> ()  [unwired: 2 in, 2 out]
                n244 = control-ref of="VISA resource name"() -> (w415:refnum<vi>)
                n245 = property on="FLOM Settings" class="Clust (strict)"("Visible"=FALSE) -> ()  [unwired: 2 in, 2 out]
                n246 = property on="SSI PR Settings" class="Clust (strict)"("Visible"=FALSE) -> ()  [unwired: 2 in, 2 out]
                n247 = property on="Masterflex 75211 Settings" class="Clust (strict)"("Visible"=FALSE) -> ()  [unwired: 2 in, 2 out]
                n248 = property on="Property Node" class="VISAName"(reference=w415, "Value"=w414) -> ()  [unwired: 1 in, 2 out]
                n249 = property on="SSI P40 Settings" class="Clust (strict)"("Visible"=FALSE) -> ()  [unwired: 2 in, 2 out]
                n250 = property on="Ismatech 3 Channel Settings" class="Clust (strict)"("Visible"=TRUE) -> ()  [unwired: 2 in, 2 out]
              }
              frame "FLOM UI-22-11" {
                n251 = property on="Ismatech" class="Clust (strict)"("Visible"=FALSE) -> ()  [unwired: 2 in, 2 out]
                n252 = property on="KNF SIMDOS Settings" class="Clust (strict)"("Visible"=FALSE) -> ()  [unwired: 2 in, 2 out]
                n253 = property on="Tacmina Settings" class="Clust (strict)"("Visible"=FALSE) -> ()  [unwired: 2 in, 2 out]
                n254 = Unbundle By Name(w425) -> ("Settings.FLOM Settings.VISA resource name"=w426:refnum<visa-resource-name>)
                n255 = property on="VICI M50 Settings" class="Clust (strict)"("Visible"=FALSE) -> ()  [unwired: 2 in, 2 out]
                n256 = property on="Masterflex" class="Clust (strict)"("Visible"=FALSE) -> ()  [unwired: 2 in, 2 out]
                n257 = property on="ASIA Pump C" class="Clust (strict)"("Visible"=FALSE) -> ()  [unwired: 2 in, 2 out]
                n258 = control-ref of="VISA resource name"() -> (w427:refnum<vi>)
                n259 = property on="FLOM Settings" class="Clust (strict)"("Visible"=TRUE) -> ()  [unwired: 2 in, 2 out]
                n260 = property on="SSI PR Settings" class="Clust (strict)"("Visible"=FALSE) -> ()  [unwired: 2 in, 2 out]
                n261 = property on="Masterflex 75211 Settings" class="Clust (strict)"("Visible"=FALSE) -> ()  [unwired: 2 in, 2 out]
                n262 = property on="Property Node" class="VISAName"(reference=w427, "Value"=w426) -> ()  [unwired: 1 in, 2 out]
                n263 = property on="SSI P40 Settings" class="Clust (strict)"("Visible"=FALSE) -> ()  [unwired: 2 in, 2 out]
                n264 = property on="Ismatech 3 Channel Settings" class="Clust (strict)"("Visible"=FALSE) -> ()  [unwired: 2 in, 2 out]
              }
              frame "Masterflex 7550-30" {
                n265 = property on="Ismatech" class="Clust (strict)"("Visible"=FALSE) -> ()  [unwired: 2 in, 2 out]
                n266 = property on="KNF SIMDOS Settings" class="Clust (strict)"("Visible"=FALSE) -> ()  [unwired: 2 in, 2 out]
                n267 = property on="Tacmina Settings" class="Clust (strict)"("Visible"=FALSE) -> ()  [unwired: 2 in, 2 out]
                n268 = Unbundle By Name(w441) -> ("Settings.Masterflex.VISA resource name"=w442:refnum<visa-resource-name>)
                n269 = property on="VICI M50 Settings" class="Clust (strict)"("Visible"=FALSE) -> ()  [unwired: 2 in, 2 out]
                n270 = property on="Masterflex" class="Clust (strict)"("Visible"=TRUE) -> ()  [unwired: 2 in, 2 out]
                n271 = property on="ASIA Pump C" class="Clust (strict)"("Visible"=FALSE) -> ()  [unwired: 2 in, 2 out]
                n272 = control-ref of="VISA resource name"() -> (w443:refnum<vi>)
                n273 = property on="FLOM Settings" class="Clust (strict)"("Visible"=FALSE) -> ()  [unwired: 2 in, 2 out]
                n274 = property on="SSI PR Settings" class="Clust (strict)"("Visible"=FALSE) -> ()  [unwired: 2 in, 2 out]
                n275 = property on="Masterflex 75211 Settings" class="Clust (strict)"("Visible"=FALSE) -> ()  [unwired: 2 in, 2 out]
                n276 = property on="Property Node" class="VISAName"(reference=w443, "Value"=w442) -> ()  [unwired: 1 in, 2 out]
                n277 = property on="SSI P40 Settings" class="Clust (strict)"("Visible"=FALSE) -> ()  [unwired: 2 in, 2 out]
                n278 = property on="Ismatech 3 Channel Settings" class="Clust (strict)"("Visible"=FALSE) -> ()  [unwired: 2 in, 2 out]
              }
              frame "VICI" {
                n279 = property on="Ismatech" class="Clust (strict)"("Visible"=FALSE) -> ()  [unwired: 2 in, 2 out]
                n280 = property on="KNF SIMDOS Settings" class="Clust (strict)"("Visible"=FALSE) -> ()  [unwired: 2 in, 2 out]
                n281 = property on="Tacmina Settings" class="Clust (strict)"("Visible"=FALSE) -> ()  [unwired: 2 in, 2 out]
                n282 = Unbundle By Name(w456) -> ("Settings.VICI Settings.VISA resource name"=w455:refnum<visa-resource-name>)
                n283 = property on="VICI M50 Settings" class="Clust (strict)"("Visible"=TRUE) -> ()  [unwired: 2 in, 2 out]
                n284 = property on="Masterflex" class="Clust (strict)"("Visible"=FALSE) -> ()  [unwired: 2 in, 2 out]
                n285 = property on="ASIA Pump C" class="Clust (strict)"("Visible"=FALSE) -> ()  [unwired: 2 in, 2 out]
                n286 = property on="FLOM Settings" class="Clust (strict)"("Visible"=FALSE) -> ()  [unwired: 2 in, 2 out]
                n287 = property on="SSI PR Settings" class="Clust (strict)"("Visible"=FALSE) -> ()  [unwired: 2 in, 2 out]
                n288 = property on="Masterflex 75211 Settings" class="Clust (strict)"("Visible"=FALSE) -> ()  [unwired: 2 in, 2 out]
                n289 = property on="VISA resource name" class="VISAName"("Value"=w455) -> ()  [unwired: 2 in, 2 out]
                n290 = property on="SSI P40 Settings" class="Clust (strict)"("Visible"=FALSE) -> ()  [unwired: 2 in, 2 out]
                n291 = property on="Ismatech 3 Channel Settings" class="Clust (strict)"("Visible"=FALSE) -> ()  [unwired: 2 in, 2 out]
              }
              frame "Default", Default {
                n292 = property on="Ismatech" class="Clust (strict)"("Visible"=FALSE) -> ()  [unwired: 2 in, 2 out]
                n293 = property on="KNF SIMDOS Settings" class="Clust (strict)"("Visible"=FALSE) -> ()  [unwired: 2 in, 2 out]
                n294 = property on="Tacmina Settings" class="Clust (strict)"("Visible"=FALSE) -> ()  [unwired: 2 in, 2 out]
                n295 = property on="VICI M50 Settings" class="Clust (strict)"("Visible"=FALSE) -> ()  [unwired: 2 in, 2 out]
                n296 = property on="Masterflex" class="Clust (strict)"("Visible"=FALSE) -> ()  [unwired: 2 in, 2 out]
                n297 = property on="ASIA Pump C" class="Clust (strict)"("Visible"=FALSE) -> ()  [unwired: 2 in, 2 out]
                n298 = property on="FLOM Settings" class="Clust (strict)"("Visible"=FALSE) -> ()  [unwired: 2 in, 2 out]
                n299 = property on="SSI PR Settings" class="Clust (strict)"("Visible"=FALSE) -> ()  [unwired: 2 in, 2 out]
                n300 = property on="Masterflex 75211 Settings" class="Clust (strict)"("Visible"=FALSE) -> ()  [unwired: 2 in, 2 out]
                n301 = property on="SSI P40 Settings" class="Clust (strict)"("Visible"=FALSE) -> ()  [unwired: 2 in, 2 out]
                n302 = property on="Ismatech 3 Channel Settings" class="Clust (strict)"("Visible"=FALSE) -> ()  [unwired: 2 in, 2 out]
              }
              frame "Tacmina QI" {
                n303 = property on="Ismatech" class="Clust (strict)"("Visible"=FALSE) -> ()  [unwired: 2 in, 2 out]
                n304 = property on="KNF SIMDOS Settings" class="Clust (strict)"("Visible"=FALSE) -> ()  [unwired: 2 in, 2 out]
                n305 = property on="Tacmina Settings" class="Clust (strict)"("Visible"=TRUE) -> ()  [unwired: 2 in, 2 out]
                n306 = property on="VICI M50 Settings" class="Clust (strict)"("Visible"=FALSE) -> ()  [unwired: 2 in, 2 out]
                n307 = property on="Masterflex" class="Clust (strict)"("Visible"=FALSE) -> ()  [unwired: 2 in, 2 out]
                n308 = property on="ASIA Pump C" class="Clust (strict)"("Visible"=FALSE) -> ()  [unwired: 2 in, 2 out]
                n309 = property on="FLOM Settings" class="Clust (strict)"("Visible"=FALSE) -> ()  [unwired: 2 in, 2 out]
                n310 = property on="SSI PR Settings" class="Clust (strict)"("Visible"=FALSE) -> ()  [unwired: 2 in, 2 out]
                n311 = property on="Masterflex 75211 Settings" class="Clust (strict)"("Visible"=FALSE) -> ()  [unwired: 2 in, 2 out]
                n312 = property on="SSI P40 Settings" class="Clust (strict)"("Visible"=FALSE) -> ()  [unwired: 2 in, 2 out]
                n313 = property on="Ismatech 3 Channel Settings" class="Clust (strict)"("Visible"=FALSE) -> ()  [unwired: 2 in, 2 out]
              }
              frame "Masterflex 75211-70" {
                n314 = property on="Ismatech" class="Clust (strict)"("Visible"=FALSE) -> ()  [unwired: 2 in, 2 out]
                n315 = property on="KNF SIMDOS Settings" class="Clust (strict)"("Visible"=FALSE) -> ()  [unwired: 2 in, 2 out]
                n316 = property on="Tacmina Settings" class="Clust (strict)"("Visible"=FALSE) -> ()  [unwired: 2 in, 2 out]
                n317 = property on="VICI M50 Settings" class="Clust (strict)"("Visible"=FALSE) -> ()  [unwired: 2 in, 2 out]
                n318 = property on="Masterflex" class="Clust (strict)"("Visible"=FALSE) -> ()  [unwired: 2 in, 2 out]
                n319 = property on="ASIA Pump C" class="Clust (strict)"("Visible"=FALSE) -> ()  [unwired: 2 in, 2 out]
                n320 = property on="FLOM Settings" class="Clust (strict)"("Visible"=FALSE) -> ()  [unwired: 2 in, 2 out]
                n321 = property on="SSI PR Settings" class="Clust (strict)"("Visible"=FALSE) -> ()  [unwired: 2 in, 2 out]
                n322 = property on="Masterflex 75211 Settings" class="Clust (strict)"("Visible"=TRUE) -> ()  [unwired: 2 in, 2 out]
                n323 = property on="SSI P40 Settings" class="Clust (strict)"("Visible"=FALSE) -> ()  [unwired: 2 in, 2 out]
                n324 = property on="Ismatech 3 Channel Settings" class="Clust (strict)"("Visible"=FALSE) -> ()  [unwired: 2 in, 2 out]
              }
              frame "KNF SIMDOS" {
                n325 = property on="Ismatech" class="Clust (strict)"("Visible"=FALSE) -> ()  [unwired: 2 in, 2 out]
                n326 = property on="KNF SIMDOS Settings" class="Clust (strict)"("Visible"=TRUE) -> ()  [unwired: 2 in, 2 out]
                n327 = property on="Tacmina Settings" class="Clust (strict)"("Visible"=FALSE) -> ()  [unwired: 2 in, 2 out]
                n328 = Unbundle By Name(w501) -> ("Settings.KNF SIMDOS Settings.VISA resource name"=w502:refnum<visa-resource-name>)
                n329 = property on="VICI M50 Settings" class="Clust (strict)"("Visible"=FALSE) -> ()  [unwired: 2 in, 2 out]
                n330 = property on="Masterflex" class="Clust (strict)"("Visible"=FALSE) -> ()  [unwired: 2 in, 2 out]
                n331 = property on="ASIA Pump C" class="Clust (strict)"("Visible"=FALSE) -> ()  [unwired: 2 in, 2 out]
                n332 = property on="FLOM Settings" class="Clust (strict)"("Visible"=FALSE) -> ()  [unwired: 2 in, 2 out]
                n333 = property on="SSI PR Settings" class="Clust (strict)"("Visible"=FALSE) -> ()  [unwired: 2 in, 2 out]
                n334 = property on="Masterflex 75211 Settings" class="Clust (strict)"("Visible"=FALSE) -> ()  [unwired: 2 in, 2 out]
                n335 = property on="VISA resource name" class="VISAName"("Value"=w502) -> ()  [unwired: 2 in, 2 out]
                n336 = property on="SSI P40 Settings" class="Clust (strict)"("Visible"=FALSE) -> ()  [unwired: 2 in, 2 out]
                n337 = property on="Ismatech 3 Channel Settings" class="Clust (strict)"("Visible"=FALSE) -> ()  [unwired: 2 in, 2 out]
              }
              frame "SSI PR/LD" {
                n338 = property on="Ismatech" class="Clust (strict)"("Visible"=FALSE) -> ()  [unwired: 2 in, 2 out]
                n339 = property on="KNF SIMDOS Settings" class="Clust (strict)"("Visible"=FALSE) -> ()  [unwired: 2 in, 2 out]
                n340 = property on="Tacmina Settings" class="Clust (strict)"("Visible"=FALSE) -> ()  [unwired: 2 in, 2 out]
                n341 = Unbundle By Name(w515) -> ("Settings.SSI PR/LD Settings.VISA resource name"=w514:refnum<visa-resource-name>)
                n342 = property on="VICI M50 Settings" class="Clust (strict)"("Visible"=FALSE) -> ()  [unwired: 2 in, 2 out]
                n343 = property on="Masterflex" class="Clust (strict)"("Visible"=FALSE) -> ()  [unwired: 2 in, 2 out]
                n344 = property on="ASIA Pump C" class="Clust (strict)"("Visible"=FALSE) -> ()  [unwired: 2 in, 2 out]
                n345 = property on="FLOM Settings" class="Clust (strict)"("Visible"=FALSE) -> ()  [unwired: 2 in, 2 out]
                n346 = property on="SSI PR Settings" class="Clust (strict)"("Visible"=TRUE) -> ()  [unwired: 2 in, 2 out]
                n347 = property on="Masterflex 75211 Settings" class="Clust (strict)"("Visible"=FALSE) -> ()  [unwired: 2 in, 2 out]
                n348 = property on="VISA resource name" class="VISAName"("Value"=w514) -> ()  [unwired: 2 in, 2 out]
                n349 = property on="SSI P40 Settings" class="Clust (strict)"("Visible"=FALSE) -> ()  [unwired: 2 in, 2 out]
                n350 = property on="Ismatech 3 Channel Settings" class="Clust (strict)"("Visible"=FALSE) -> ()  [unwired: 2 in, 2 out]
              }
              frame "SSI P40" {
                n351 = property on="Ismatech" class="Clust (strict)"("Visible"=FALSE) -> ()  [unwired: 2 in, 2 out]
                n352 = property on="KNF SIMDOS Settings" class="Clust (strict)"("Visible"=FALSE) -> ()  [unwired: 2 in, 2 out]
                n353 = property on="Tacmina Settings" class="Clust (strict)"("Visible"=FALSE) -> ()  [unwired: 2 in, 2 out]
                n354 = Unbundle By Name(w528) -> ("Settings.SSI PR/LD Settings.VISA resource name"=w527:refnum<visa-resource-name>)
                n355 = property on="VICI M50 Settings" class="Clust (strict)"("Visible"=FALSE) -> ()  [unwired: 2 in, 2 out]
                n356 = property on="Masterflex" class="Clust (strict)"("Visible"=FALSE) -> ()  [unwired: 2 in, 2 out]
                n357 = property on="ASIA Pump C" class="Clust (strict)"("Visible"=FALSE) -> ()  [unwired: 2 in, 2 out]
                n358 = property on="FLOM Settings" class="Clust (strict)"("Visible"=FALSE) -> ()  [unwired: 2 in, 2 out]
                n359 = property on="SSI PR Settings" class="Clust (strict)"("Visible"=FALSE) -> ()  [unwired: 2 in, 2 out]
                n360 = property on="Masterflex 75211 Settings" class="Clust (strict)"("Visible"=FALSE) -> ()  [unwired: 2 in, 2 out]
                n361 = property on="VISA resource name" class="VISAName"("Value"=w527) -> ()  [unwired: 2 in, 2 out]
                n362 = property on="SSI P40 Settings" class="Clust (strict)"("Visible"=TRUE) -> ()  [unwired: 2 in, 2 out]
                n363 = property on="Ismatech 3 Channel Settings" class="Clust (strict)"("Visible"=FALSE) -> ()  [unwired: 2 in, 2 out]
              }
              frame "ASIA Type C" {
                n364 = property on="Ismatech" class="Clust (strict)"("Visible"=FALSE) -> ()  [unwired: 2 in, 2 out]
                n365 = property on="KNF SIMDOS Settings" class="Clust (strict)"("Visible"=FALSE) -> ()  [unwired: 2 in, 2 out]
                n366 = property on="Tacmina Settings" class="Clust (strict)"("Visible"=FALSE) -> ()  [unwired: 2 in, 2 out]
                n367 = Unbundle By Name(w540) -> ("Settings.ASIA Pump C.ASIA Pump #"=w543:i32)
                n368 = Unbundle By Name(w540) -> ("Settings.ASIA Pump C.channel"=w542:i32)
                n369 = property on="VICI M50 Settings" class="Clust (strict)"("Visible"=FALSE) -> ()  [unwired: 2 in, 2 out]
                n370 = property on="Masterflex" class="Clust (strict)"("Visible"=FALSE) -> ()  [unwired: 2 in, 2 out]
                n371 = property on="ASIA Pump C" class="Clust (strict)"("Visible"=TRUE) -> ()  [unwired: 2 in, 2 out]
                n372 = control-ref of="channel"() -> (w541:refnum<vi>)
                n373 = control-ref of="ASIA Pump #"() -> (w544:refnum<vi>)
                n374 = property on="FLOM Settings" class="Clust (strict)"("Visible"=FALSE) -> ()  [unwired: 2 in, 2 out]
                n375 = property on="SSI PR Settings" class="Clust (strict)"("Visible"=FALSE) -> ()  [unwired: 2 in, 2 out]
                n376 = property on="Masterflex 75211 Settings" class="Clust (strict)"("Visible"=FALSE) -> ()  [unwired: 2 in, 2 out]
                n377 = property on="Property Node" class="DigNum (strict)"(reference=w544, "Value"=w543) -> ()  [unwired: 1 in, 2 out]
                n378 = property on="Property Node" class="DigNum (strict)"(reference=w541, "Value"=w542) -> ()  [unwired: 1 in, 2 out]
                n379 = property on="SSI P40 Settings" class="Clust (strict)"("Visible"=FALSE) -> ()  [unwired: 2 in, 2 out]
                n380 = property on="Ismatech 3 Channel Settings" class="Clust (strict)"("Visible"=FALSE) -> ()  [unwired: 2 in, 2 out]
              }
            }
          }
          event Value Change {
            n381 = event-data() -> ("OldVal"=w551:refnum<visa-resource-name>)  [unwired: 1 in]
            n382 = local read "Settings Dialog"() -> (w554:T17)
            n383 = Unbundle By Name(w554) -> ("SSI PR/LD Settings"=w548:T13)
            n384 = VISA Close(VISA resource name=w551) -> (error out=w547:errorcluster)  [unwired: 1 in]
            n385 = call "Initialize.vi"("error in (no error)"=w547, "SSI PR Settings In"=w548) -> ("Initialized"=w545:bool, "SSI PR Settings Out"=w546:T13)  [unwired: 6 in, 2 out]
            n386 = case shown="False" w545 {
              tunnel: w546 -> [_ w559]
              tunnel: w553 -> [w558 w563]
              tunnel: [w558 w562] -> w552
              frame False {
                n387 = control-ref of="OK Button"() -> (w556:refnum<vi>)
                n388 = property on="Property Node" class="Bool"(reference=w556, "DisabledEnum"=T22."Disabled and Grayed Out" ("Disabled")) -> ()  [unwired: 1 in, 2 out]
                n389 = One Button Dialog(message="No Pump Connected") -> ()  [unwired: 1 in, 1 out]
              }
              frame True {
                n390 = Bundle By Name(cluster=w563, "Settings.SSI PR/LD Settings"=w559) -> (w562:T18)
                n391 = control-ref of="OK Button"() -> (w560:refnum<vi>)
                n392 = property on="Property Node" class="Bool"(reference=w560, "DisabledEnum"=T22."Enabled" ("Disabled")) -> ()  [unwired: 1 in, 2 out]
              }
            }
          }
          event Value Change {
            n393 = event-data() -> ("OldVal"=w570:refnum<visa-resource-name>)  [unwired: 1 in]
            n394 = local read "Settings Dialog"() -> (w573:T17)
            n395 = Unbundle By Name(w573) -> ("SSI P40 Settings"=w567:T15)
            n396 = VISA Close(VISA resource name=w570) -> (error out=w566:errorcluster)  [unwired: 1 in]
            n397 = call "Initialize P40.vi"("error in (no error)"=w566, "SSI P40 Settings In"=w567) -> ("Initialized"=w564:bool, "SSI P40 Settings Out"=w565:T15)  [unwired: 6 in, 2 out]
            n398 = case shown="False" w564 {
              tunnel: w565 -> [_ w578]
              tunnel: w572 -> [w577 w582]
              tunnel: [w577 w581] -> w571
              frame False {
                n399 = control-ref of="OK Button"() -> (w575:refnum<vi>)
                n400 = property on="Property Node" class="Bool"(reference=w575, "DisabledEnum"=T22."Disabled and Grayed Out" ("Disabled")) -> ()  [unwired: 1 in, 2 out]
                n401 = One Button Dialog(message="No Pump Connected") -> ()  [unwired: 1 in, 1 out]
              }
              frame True {
                n402 = Bundle By Name(cluster=w582, "Settings.SSI PR/LD Settings"=w578) -> (w581:T18)
                n403 = control-ref of="OK Button"() -> (w579:refnum<vi>)
                n404 = property on="Property Node" class="Bool"(reference=w579, "DisabledEnum"=T22."Enabled" ("Disabled")) -> ()  [unwired: 1 in, 2 out]
              }
            }
          }
          event Value Change {
            n405 = event-data() -> ()  [unwired: 1 in, 1 out]
            n406 = local read "Settings Dialog"() -> (w586:T17)
            n407 = Unbundle By Name(w586) -> ("VICI M50 Settings"=w585:T11)
            n408 = case shown="True" w583 {
              tunnel: [w589 w594] -> w588
              tunnel: w587 -> [w589 w593]
              tunnel: w585 -> [_ w591]
              frame False {
              }
              frame True {
                n409 = call "Initialize.vi"("VICI Settings"=w591) -> ("Initialized"=w590:bool, "VICI Settings"=w592:T11)  [unwired: 7 in, 2 out]
                n410 = case shown="False" w590 {
                  tunnel: [w598 w603] -> w594
                  tunnel: w593 -> [w598 w602]
                  tunnel: w592 -> [_ w599]
                  frame False {
                    n411 = control-ref of="OK Button"() -> (w596:refnum<vi>)
                    n412 = property on="Property Node" class="Bool"(reference=w596, "DisabledEnum"=T22."Disabled and Grayed Out" ("Disabled")) -> ()  [unwired: 1 in, 2 out]
                    n413 = One Button Dialog(message="No Pump Connected") -> ()  [unwired: 1 in, 1 out]
                  }
                  frame True {
                    n414 = Bundle By Name(cluster=w602, "Settings.VICI Settings"=w599) -> (w603:T18)
                    n415 = control-ref of="OK Button"() -> (w600:refnum<vi>)
                    n416 = property on="Property Node" class="Bool"(reference=w600, "DisabledEnum"=T22."Enabled" ("Disabled")) -> ()  [unwired: 1 in, 2 out]
                  }
                }
              }
            }
          }
          event Value Change {
            n417 = event-data() -> ("OldVal"=w606:refnum<visa-resource-name>)  [unwired: 1 in]
            n418 = local read "Settings Dialog"() -> (w609:T17)
            n419 = Unbundle By Name(w609) -> ("VICI M50 Settings"=w608:T11)
            n420 = VISA Close(VISA resource name=w606) -> (error out=w607:errorcluster)  [unwired: 1 in]
            n421 = case shown="True" w604 {
              tunnel: [w612 w618] -> w611
              tunnel: w610 -> [w612 w617]
              tunnel: w608 -> [_ w615]
              tunnel: w607 -> [_ w614]
              frame False {
              }
              frame True {
                n422 = call "Initialize.vi"("error in (no error)"=w614, "VICI Settings"=w615) -> ("Initialized"=w613:bool, "VICI Settings"=w616:T11)  [unwired: 6 in, 2 out]
                n423 = case shown="True" w613 {
                  tunnel: [w622 w627] -> w618
                  tunnel: w617 -> [w622 w626]
                  tunnel: w616 -> [_ w623]
                  frame False {
                    n424 = control-ref of="OK Button"() -> (w620:refnum<vi>)
                    n425 = property on="Property Node" class="Bool"(reference=w620, "DisabledEnum"=T22."Disabled and Grayed Out" ("Disabled")) -> ()  [unwired: 1 in, 2 out]
                    n426 = One Button Dialog(message="No Pump Connected") -> ()  [unwired: 1 in, 1 out]
                  }
                  frame True {
                    n427 = Bundle By Name(cluster=w626, "Settings.VICI Settings"=w623) -> (w627:T18)
                    n428 = control-ref of="OK Button"() -> (w624:refnum<vi>)
                    n429 = property on="Property Node" class="Bool"(reference=w624, "DisabledEnum"=T22."Enabled" ("Disabled")) -> ()  [unwired: 1 in, 2 out]
                  }
                }
              }
            }
          }
        }
      }
      n430 = Unbundle By Name(w19) -> ("Settings.PID 2 Parameters.Input Device"=w18:T5)
      n431 = Not Equal?(x=PID_Input_Enum."Default", y=w18) -> (x != y?=w16:bool)
      n432 = case "Load settings if there are any written" shown="True" w16 {
        tunnel: w19 -> [_ w43]
        frame False {
        }
        frame True {
          n433 = Unbundle By Name(w43) -> ("Settings"=w52:T20)
          n434 = Unbundle By Name(w52) -> ("Cycle Period"=w53:dbl, "Ismatech"=w54:T1, "Masterflex"=w44:T2, "Mettler"=w45:T3, "Bronkhorst M13 Flow Meter"=w46:T4, "PID 2 Parameters"=w47:T21, "Bronkhorst M14 Settings"=w30:T7, "output range"=w31:cluster{"output high":dbl, "output low":dbl}, "Tacmina Settings"=w41:T8, "KNF SIMDOS Settings"=w40:T9, "ASIA Pump C"=w39:T10, "VICI Settings"=w38:T11, "FLOM Settings"=w37:T12, "SSI PR/LD Settings"=w36:T13, "Masterflex 75211 Settings"=w35:T14, "SSI P40 Settings"=w34:T15, "Ismatech 3 Channel Settings"=w33:T16)
          n435 = Unbundle(w47) -> ("Input Device"=w50:T5, "Output Device"=w51:T6, "PID gains"=w48:T24)  [unwired: 1 out]
          n436 = local read "Settings Dialog"() -> (w42:T17)
          n437 = Bundle("Input Device"=w50, "Output Device"=w51, "PID gains"=w48) -> (w49:T23)  [unwired: 1 in]
          n438 = Bundle By Name(cluster=w42, "Cycle Period"=w53, "Ismatech"=w54, "Masterflex"=w44, "Mettler"=w45, "Bronkhorst M13 Settings"=w46, "PID 2 Parameters"=w49, "Bronkhorst M14 Settings"=w30, "PID2 Range"=w31, "Tacmina Settings"=w41, "KNF SIMDOS Settings"=w40, "ASIA Pump C"=w39, "VICI M50 Settings"=w38, "FLOM Settings"=w37, "SSI PR/LD Settings"=w36, "Masterflex 75211 Settings"=w35, "SSI P40 Settings"=w34, "Ismatech 3 Channel Settings"=w33) -> (w32:T17)
          n439 = local write "Settings Dialog"(w32) -> ()
          n440 = property on="Settings Dialog" class="Clust (strict)"("Val(Sgnl)"=w32) -> ()  [unwired: 2 in, 2 out]
          n441 = property on="Input Device" class="Enum (strict)"("Val(Sgnl)"=w50) -> ()  [unwired: 2 in, 2 out]
          n442 = property on="Output Device" class="Enum (strict)"("Val(Sgnl)"=w51) -> ()  [unwired: 2 in, 2 out]
        }
      }
    }
    frame Error {
    }
  }
  "UI Refresh Needed?" <- w13
  "error out" <- w14
  "Feed Module Config out" <- w10
  "Cancelled?" <- w12
